vi "ConvertTextBasedCodeToLabVIEW_CreateClasses.vi"(0 "Classes":T11[](array[typedef])=[{"ClassName"="Program", "AccessScope"=enum."public", "Modifiers"=[], "ClassDocumentation"="", "Methods"=[{"ReturnType"={"Name"="", "DataType"=enum."void", "ArrayDim"=0, "CtrlPath"=path "", "DataTypeString"="void", "AccessScope"=enum."public", "InitialData"=variant(string "")}, "MethodName"="Main", "AccessScope"=enum."public", "Modifiers"=[enum."static"], "MethodDocumentation"="", "MethodContent"="public static void Main(string[] args)\n        {\n            // Create a subject and the observable, inject the subject into the observable\n            Subject subject = new Subject();\n            SubjectObservable observable = new SubjectObservable(subject);\n\n            //Create two observers\n            SubjectObserver zeus = new SubjectObserver(observable, \"Zeus\");\n            SubjectObserver ares = new SubjectObserver(observable, \"Ares\");\n            \n            // Run a loop and trigger the observer\n            for (int i = 0; i < 5; i++)\n            {\n                Console.WriteLine(\"Counter: \" + subject.Counter);\n                observable.inspectSubject();\n\n            }\n\n            Console.ReadLine();\n        }", "MethodArguments"=[{"Name"="args", "DataType"=enum."STRING", "ArrayDim"=1, "CtrlPath"=path "", "DataTypeString"="string[]", "AccessScope"=enum."public", "InitialData"=variant(string "")}], "GetProperty"={"Active"=FALSE, "AccessScope"=enum."public", "Code"=""}, "SetProperty"={"Active"=FALSE, "AccessScope"=enum."public", "Code"=""}}], "ParentClasses"=[], "ClassType"=enum."Class", "Owner"="Test", "OwnerType"=enum."Package/NameSpace", "Generics"=[], "Attributes"=[{"Name"="MyUINT8", "DataType"=enum."UINT8", "ArrayDim"=0, "CtrlPath"=path "", "DataTypeString"="", "AccessScope"=enum."public", "InitialData"=variant}], "Enums"=[{"Name"="MyEnum", "AccessScope"=enum."public", "Modifiers"=[], "Items"=["A1", "A2"], "Documentation"="My Enum Doc"}], "Structs"=[{"Name"="MyStruct", "AccessScope"=enum."public", "Modifiers"=[], "Items"=[{"Name"="MyObject", "DataType"=enum."LabVIEW Class", "ArrayDim"=1, "CtrlPath"=path "", "DataTypeString"="Program", "AccessScope"=enum."public", "InitialData"=variant}, {"Name"="Sträng", "DataType"=enum."STRING", "ArrayDim"=0, "CtrlPath"=path "", "DataTypeString"="", "AccessScope"=enum."public", "InitialData"=variant}], "Documentation"="Struct Doc"}]}, {"ClassName"="Subject", "AccessScope"=enum."public", "Modifiers"=[], "ClassDocumentation"="Class Subject - It has a counter object that increases everytime you inspect it", "Methods"=[{"ReturnType"={"Name"="", "DataType"=enum."INT32", "ArrayDim"=0, "CtrlPath"=path "", "DataTypeString"="int", "AccessScope"=enum."public", "InitialData"=variant(string "")}, "MethodName"="Counter", "AccessScope"=enum."public", "Modifiers"=[], "MethodDocumentation"="", "MethodContent"="public int Counter\n        {\n            get\n            {\n                return ++_counter;\n            }\n        }", "MethodArguments"=[], "GetProperty"={"Active"=TRUE, "AccessScope"=enum."public", "Code"="return ++_counter;"}, "SetProperty"={"Active"=FALSE, "AccessScope"=enum."public", "Code"=""}}], "ParentClasses"=[], "ClassType"=enum."Class", "Owner"="Test", "OwnerType"=enum."Package/NameSpace", "Generics"=[], "Attributes"=[{"Name"="_counter", "DataType"=enum."INT32", "ArrayDim"=0, "CtrlPath"=path "", "DataTypeString"="int", "AccessScope"=enum."private", "InitialData"=variant(string "")}], "Enums"=[], "Structs"=[]}, {"ClassName"="SubjectObservable", "AccessScope"=enum."public", "Modifiers"=[], "ClassDocumentation"="Class Subject Observable - The observable object that observes the subject and notifies the observers", "Methods"=[{"ReturnType"={"Name"="", "DataType"=enum."LabVIEW Object", "ArrayDim"=0, "CtrlPath"=path "", "DataTypeString"="SubjectObservable", "AccessScope"=enum."public", "InitialData"=variant(string "")}, "MethodName"="SubjectObservable", "AccessScope"=enum."public", "Modifiers"=[], "MethodDocumentation"="Accept a subject instance which we shall observe", "MethodContent"="public SubjectObservable(Subject subject)\n        {\n            _subjectObservers = new List<IObserver<Subject>>();\n            _subject = subject;\n\n        }", "MethodArguments"=[{"Name"="subject", "DataType"=enum."LabVIEW Object", "ArrayDim"=0, "CtrlPath"=path "", "DataTypeString"="Subject", "AccessScope"=enum."public", "InitialData"=variant(string "")}], "GetProperty"={"Active"=FALSE, "AccessScope"=enum."public", "Code"=""}, "SetProperty"={"Active"=FALSE, "AccessScope"=enum."public", "Code"=""}}, {"ReturnType"={"Name"="", "DataType"=enum."Other", "ArrayDim"=0, "CtrlPath"=path "", "DataTypeString"="IDisposable", "AccessScope"=enum."public", "InitialData"=variant(string "")}, "MethodName"="Subscribe", "AccessScope"=enum."public", "Modifiers"=[], "MethodDocumentation"="This method allows the observers to attach themselves. It returns a disposer object to the observer\nwhich the observer can utilize to unsubscribe", "MethodContent"="public IDisposable Subscribe(IObserver<Subject> observer)\n        {\n            if (!_subjectObservers.Contains(observer))\n            {\n                _subjectObservers.Add(observer);\n            }\n\n            return new Disposer(_subjectObservers, observer);\n        }", "MethodArguments"=[{"Name"="observer", "DataType"=enum."Other", "ArrayDim"=0, "CtrlPath"=path "", "DataTypeString"="IObserver<Subject>", "AccessScope"=enum."public", "InitialData"=variant(string "")}], "GetProperty"={"Active"=FALSE, "AccessScope"=enum."public", "Code"=""}, "SetProperty"={"Active"=FALSE, "AccessScope"=enum."public", "Code"=""}}, {"ReturnType"={"Name"="", "DataType"=enum."void", "ArrayDim"=0, "CtrlPath"=path "", "DataTypeString"="void", "AccessScope"=enum."public", "InitialData"=variant(string "")}, "MethodName"="inspectSubject", "AccessScope"=enum."public", "Modifiers"=[enum."event"], "MethodDocumentation"="This method is used to inspect the subject over time. Usually used with a timer or an event", "MethodContent"="event\n        public void inspectSubject()\n        {\n            foreach (IObserver<Subject> observer in _subjectObservers)\n            {\n                observer.OnNext(_subject);\n            }\n        }", "MethodArguments"=[], "GetProperty"={"Active"=FALSE, "AccessScope"=enum."public", "Code"=""}, "SetProperty"={"Active"=FALSE, "AccessScope"=enum."public", "Code"=""}}], "ParentClasses"=[{"ClassName"="IObservable", "ClassType"=enum."Undefined"}], "ClassType"=enum."Class", "Owner"="Test", "OwnerType"=enum."Package/NameSpace", "Generics"=["Subject"], "Attributes"=[{"Name"="_subjectObservers", "DataType"=enum."Other", "ArrayDim"=1, "CtrlPath"=path "", "DataTypeString"="IObserver<Subject>", "AccessScope"=enum."private", "InitialData"=variant(string "")}, {"Name"="_subject", "DataType"=enum."LabVIEW Object", "ArrayDim"=0, "CtrlPath"=path "", "DataTypeString"="Subject", "AccessScope"=enum."private", "InitialData"=variant(string "")}], "Enums"=[], "Structs"=[]}, {"ClassName"="SubjectObserver", "AccessScope"=enum."public", "Modifiers"=[], "ClassDocumentation"="Class Subject Observer - The object that attaches itself to a observable and recieves notifications", "Methods"=[{"ReturnType"={"Name"="", "DataType"=enum."LabVIEW Object", "ArrayDim"=0, "CtrlPath"=path "", "DataTypeString"="SubjectObserver", "AccessScope"=enum."public", "InitialData"=variant(string "")}, "MethodName"="SubjectObserver", "AccessScope"=enum."public", "Modifiers"=[], "MethodDocumentation"="", "MethodContent"="public SubjectObserver(IObservable<Subject> provider, string instanceName)\n        {\n            if (provider != null)\n            {\n                _disposer = provider.Subscribe(this);\n                _instaceName = instanceName;\n            }\n        }", "MethodArguments"=[{"Name"="provider", "DataType"=enum."Other", "ArrayDim"=0, "CtrlPath"=path "", "DataTypeString"="IObservable<Subject>", "AccessScope"=enum."public", "InitialData"=variant(string "")}, {"Name"="instanceName", "DataType"=enum."STRING", "ArrayDim"=0, "CtrlPath"=path "", "DataTypeString"="string", "AccessScope"=enum."public", "InitialData"=variant(string "")}], "GetProperty"={"Active"=FALSE, "AccessScope"=enum."public", "Code"=""}, "SetProperty"={"Active"=FALSE, "AccessScope"=enum."public", "Code"=""}}, {"ReturnType"={"Name"="", "DataType"=enum."void", "ArrayDim"=0, "CtrlPath"=path "", "DataTypeString"="void", "AccessScope"=enum."public", "InitialData"=variant(string "")}, "MethodName"="OnNext", "AccessScope"=enum."public", "Modifiers"=[], "MethodDocumentation"="The observable invokes this method to pass the Subject object to the observer", "MethodContent"="public void OnNext(Subject value)\n        {\n            Console.WriteLine(\"[\" + _instaceName + \"] \" + value.Counter);\n        }", "MethodArguments"=[{"Name"="value", "DataType"=enum."LabVIEW Object", "ArrayDim"=0, "CtrlPath"=path "", "DataTypeString"="Subject", "AccessScope"=enum."public", "InitialData"=variant(string "")}], "GetProperty"={"Active"=FALSE, "AccessScope"=enum."public", "Code"=""}, "SetProperty"={"Active"=FALSE, "AccessScope"=enum."public", "Code"=""}}, {"ReturnType"={"Name"="", "DataType"=enum."void", "ArrayDim"=0, "CtrlPath"=path "", "DataTypeString"="void", "AccessScope"=enum."public", "InitialData"=variant(string "")}, "MethodName"="OnCompleted", "AccessScope"=enum."public", "Modifiers"=[], "MethodDocumentation"="Usually called when a transmission is complete. Not implemented.", "MethodContent"="public void OnCompleted()\n        {\n            throw new NotImplementedException();\n        }", "MethodArguments"=[], "GetProperty"={"Active"=FALSE, "AccessScope"=enum."public", "Code"=""}, "SetProperty"={"Active"=FALSE, "AccessScope"=enum."public", "Code"=""}}, {"ReturnType"={"Name"="", "DataType"=enum."void", "ArrayDim"=0, "CtrlPath"=path "", "DataTypeString"="void", "AccessScope"=enum."public", "InitialData"=variant(string "")}, "MethodName"="OnError", "AccessScope"=enum."public", "Modifiers"=[], "MethodDocumentation"="Usually called when there was an error. Didn't implement.", "MethodContent"="public void OnError(Exception error)\n        {\n            throw new NotImplementedException();\n        }", "MethodArguments"=[{"Name"="error", "DataType"=enum."Other", "ArrayDim"=0, "CtrlPath"=path "", "DataTypeString"="Exception", "AccessScope"=enum."public", "InitialData"=variant(string "")}], "GetProperty"={"Active"=FALSE, "AccessScope"=enum."public", "Code"=""}, "SetProperty"={"Active"=FALSE, "AccessScope"=enum."public", "Code"=""}}, {"ReturnType"={"Name"="", "DataType"=enum."void", "ArrayDim"=0, "CtrlPath"=path "", "DataTypeString"="void", "AccessScope"=enum."public", "InitialData"=variant(string "")}, "MethodName"="Dispose", "AccessScope"=enum."public", "Modifiers"=[], "MethodDocumentation"="Invoke the disposer recieved from the observable. This will unsubscribe", "MethodContent"="public void Dispose()\n        {\n            _disposer.Dispose();\n        }", "MethodArguments"=[], "GetProperty"={"Active"=FALSE, "AccessScope"=enum."public", "Code"=""}, "SetProperty"={"Active"=FALSE, "AccessScope"=enum."public", "Code"=""}}], "ParentClasses"=[{"ClassName"="IObserver", "ClassType"=enum."Undefined"}], "ClassType"=enum."Class", "Owner"="Test", "OwnerType"=enum."Package/NameSpace", "Generics"=["Subject"], "Attributes"=[{"Name"="_disposer", "DataType"=enum."Other", "ArrayDim"=0, "CtrlPath"=path "", "DataTypeString"="IDisposable", "AccessScope"=enum."private", "InitialData"=variant(string "")}, {"Name"="_instaceName", "DataType"=enum."STRING", "ArrayDim"=0, "CtrlPath"=path "", "DataTypeString"="string", "AccessScope"=enum."private", "InitialData"=variant(string "")}], "Enums"=[], "Structs"=[]}, {"ClassName"="Disposer", "AccessScope"=enum."private", "Modifiers"=[], "ClassDocumentation"="Private class Disposer: Implements the IDisposable. Observable returns an instance to the observer for easy unsubscription\nprivate", "Methods"=[{"ReturnType"={"Name"="", "DataType"=enum."LabVIEW Object", "ArrayDim"=0, "CtrlPath"=path "", "DataTypeString"="Disposer", "AccessScope"=enum."public", "InitialData"=variant(string "")}, "MethodName"="Disposer", "AccessScope"=enum."public", "Modifiers"=[], "MethodDocumentation"="", "MethodContent"="public Disposer(List<IObserver<Subject>> _subObservers, IObserver<Subject> observer)\n            {\n                _subjectObservers = _subObservers;\n                _observer = observer;\n            }", "MethodArguments"=[{"Name"="_subObservers", "DataType"=enum."Other", "ArrayDim"=1, "CtrlPath"=path "", "DataTypeString"="IObserver<Subject>", "AccessScope"=enum."public", "InitialData"=variant(string "")}, {"Name"="observer", "DataType"=enum."Other", "ArrayDim"=0, "CtrlPath"=path "", "DataTypeString"="IObserver<Subject>", "AccessScope"=enum."public", "InitialData"=variant(string "")}], "GetProperty"={"Active"=FALSE, "AccessScope"=enum."public", "Code"=""}, "SetProperty"={"Active"=FALSE, "AccessScope"=enum."public", "Code"=""}}, {"ReturnType"={"Name"="", "DataType"=enum."void", "ArrayDim"=0, "CtrlPath"=path "", "DataTypeString"="void", "AccessScope"=enum."public", "InitialData"=variant(string "")}, "MethodName"="Dispose", "AccessScope"=enum."public", "Modifiers"=[], "MethodDocumentation"="", "MethodContent"="public void Dispose()\n            {\n                if (_subjectObservers.Contains(_observer))\n                {\n                    _subjectObservers.Remove(_observer);\n                }\n            }", "MethodArguments"=[], "GetProperty"={"Active"=FALSE, "AccessScope"=enum."public", "Code"=""}, "SetProperty"={"Active"=FALSE, "AccessScope"=enum."public", "Code"=""}}], "ParentClasses"=[{"ClassName"="IDisposable", "ClassType"=enum."Undefined"}], "ClassType"=enum."Class", "Owner"="SubjectObservable", "OwnerType"=enum."Class", "Generics"=[], "Attributes"=[{"Name"="_subjectObservers", "DataType"=enum."Other", "ArrayDim"=1, "CtrlPath"=path "", "DataTypeString"="IObserver<Subject>", "AccessScope"=enum."private", "InitialData"=variant(string "")}, {"Name"="_observer", "DataType"=enum."Other", "ArrayDim"=0, "CtrlPath"=path "", "DataTypeString"="IObserver<Subject>", "AccessScope"=enum."private", "InitialData"=variant(string "")}], "Enums"=[], "Structs"=[]}], 1 "TopFolder":path=path "D:/Temp", 2 "InterfacesThatShouldBeConvertedToClasses":string[](array[string]), 3 "Options":T7={"ClassProvider"=enum."LabVIEW Native(By value)", "PropertyMethodType"=enum."PropertyMethod", "Pattern type"=2} {"Pattern type" items=["4x4x4", "5x6x5", "6x8x6"]}, 5 "MissingItems":T17[](array[typedef])=[{"Item"="IObservable", "Options"=["Select action to handle missing type", "Create stub code as class", "Create stub code as interface by VI Server", "Remove dependency to this type"], "Icons"=[enum."?", enum."Add", enum."Add", enum."Delete"], "Index"=2}, {"Item"="IDisposable", "Options"=["Select action to handle missing type", "Create stub code as class", "Create stub code as interface by VI Server", "Remove dependency to this type"], "Icons"=[enum."?", enum."Add", enum."Add", enum."Delete"], "Index"=1}, {"Item"="IObserver", "Options"=["Select action to handle missing type", "Create stub code as class", "Create stub code as interface by VI Server", "Remove dependency to this type"], "Icons"=[enum."?", enum."Add", enum."Add", enum."Delete"], "Index"=2}, {"Item"="Exception", "Options"=["Select action to handle missing type", "Create stub code as class", "Remove dependency to this type"], "Icons"=[enum."?", enum."Add", enum."Delete"], "Index"=2}], 7 "BetterNames":bool, 9 "ExistingClassFolders":path[](array[path]), 11 "error in (no error)":errorcluster, 12 "ProgressTextRef":refnum<vi>, 13 "StructsOusideClass":T1[](array[typedef]), 14 "EnumsOusideClass":T6[](array[typedef])) -> (15 "error out":errorcluster)   [LabVIEW 2016]
uses:
  <resource>/Framework/Providers/Open_GDS/ClassProviders/Common/ConvertTextToLv_SubVIs/ConvertTextBasedCodeToLabVIEW_MissingType.ctl
  <resource>/Framework/Providers/Open_GDS/ClassProviders/Common/ConvertTextToLv_SubVIs/ConvertTextBasedCodeToLabVIEW_MissingTypeIconType.ctl
  <resource>/Framework/Providers/Open_GDS/ClassProviders/Common/String/GDSString_ClassDescriptionType.ctl
  <resource>/Framework/Providers/Open_GDS/ClassProviders/Common/String/GDSString_AccessScopeModifierType.ctl
  <resource>/Framework/Providers/Open_GDS/ClassProviders/Common/String/GDSString_ModifierType.ctl
  <resource>/Framework/Providers/Open_GDS/ClassProviders/Common/String/GDSString_MethodDescriptionType.ctl
  <resource>/Framework/Providers/Open_GDS/ClassProviders/Common/CommonVIs/CommonVIs_AttributeType.ctl
  <resource>/Framework/Providers/Open_GDS/ClassProviders/Common/CommonVIs/CommonVIs_AttributeDataType.ctl
  <resource>/Framework/Providers/Open_GDS/ClassProviders/Common/CommonVIs/CommonVIs_PropertyType.ctl
  <resource>/Framework/Providers/Open_GDS/ClassProviders/Common/String/GDSString_ClassParentType.ctl
  <resource>/Framework/Providers/Open_GDS/ClassProviders/Common/String/GDSString_ClassType.ctl
  <resource>/Framework/Providers/Open_GDS/ClassProviders/Common/String/GDSString_ClassOwnerType.ctl
  <resource>/Framework/Providers/Open_GDS/ClassProviders/Common/CommonVIs/CommonVIs_EnumType.ctl
  <resource>/Framework/Providers/Open_GDS/ClassProviders/Common/CommonVIs/CommonVIs_StructType.ctl
  <resource>/Framework/Providers/Open_GDS/ClassProviders/Common/ConvertTextToLv_SubVIs/ConvertTextBasedCodeToLabVIEW_CreateClassesOption.ctl
  <resource>/Framework/Providers/Open_GDS/API/GDSAPI_SubVIs/GDSAPI_ClassProviderType.ctl
  <resource>/Framework/Providers/Open_GDS/API/GDSAPI_SubVIs/GDSAPI_PropertyMethodType.ctl
  <resource>/Framework/Providers/Open_GDS/ClassProviders/Common/ScriptingFunctions/Scripting_ConnectorPanePatternType.ctl
  <resource>/Framework/Providers/Open_GDS/ClassProviders/Common/CommonVIs/CommonVIs_ClassNamePathType.ctl
  <resource>/Framework/Providers/Open_GDS/API/GDSAPI_SubVIs/GDSAPI_SetClassOptionsAction.ctl
  <resource>/Framework/Providers/Open_GDS/ClassProviders/Common/ConvertTextToLv_SubVIs/ConvertTextBasedCodeToLabVIEW_MissingTypeOptions.ctl
  <resource>/Framework/Providers/Open_GDS/API/GDSAPI_CreateClassType.ctl
  <resource>/Framework/Providers/Open_GDS/API/GDSAPI_SubVIs/GDSAPI_ClassTemplateType.ctl
  <resource>/Framework/Providers/Open_GDS/API/GDSAPI_SubVIs/GDSAPI_ProjectIconType.ctl
panel:
  out "ClassesOut":T11[](array[typedef])=[{"ClassName"="Program", "AccessScope"=enum."public", "Modifiers"=[], "ClassDocumentation"="", "Methods"=[{"ReturnType"={"Name"="", "DataType"=enum."void", "ArrayDim"=0, "CtrlPath"=path "", "DataTypeString"="void", "AccessScope"=enum."public", "InitialData"=variant(string "")}, "MethodName"="Main", "AccessScope"=enum."public", "Modifiers"=[enum."static"], "MethodDocumentation"="", "MethodContent"="public static void Main(string[] args)\n        {\n            // Create a subject and the observable, inject the subject into the observable\n            Subject subject = new Subject();\n            SubjectObservable observable = new SubjectObservable(subject);\n\n            //Create two observers\n            SubjectObserver zeus = new SubjectObserver(observable, \"Zeus\");\n            SubjectObserver ares = new SubjectObserver(observable, \"Ares\");\n            \n            // Run a loop and trigger the observer\n            for (int i = 0; i < 5; i++)\n            {\n                Console.WriteLine(\"Counter: \" + subject.Counter);\n                observable.inspectSubject();\n\n            }\n\n            Console.ReadLine();\n        }", "MethodArguments"=[{"Name"="args", "DataType"=enum."STRING", "ArrayDim"=1, "CtrlPath"=path "", "DataTypeString"="string[]", "AccessScope"=enum."public", "InitialData"=variant(string "")}], "GetProperty"={"Active"=FALSE, "AccessScope"=enum."public", "Code"=""}, "SetProperty"={"Active"=FALSE, "AccessScope"=enum."public", "Code"=""}}], "ParentClasses"=[], "ClassType"=enum."Class", "Owner"="Test", "OwnerType"=enum."Package/NameSpace", "Generics"=[], "Attributes"=[{"Name"="MyUINT8", "DataType"=enum."UINT8", "ArrayDim"=0, "CtrlPath"=path "", "DataTypeString"="", "AccessScope"=enum."public", "InitialData"=variant}], "Enums"=[{"Name"="MyEnum", "AccessScope"=enum."public", "Modifiers"=[], "Items"=["A1", "A2"], "Documentation"="My Enum Doc"}], "Structs"=[{"Name"="MyStruct", "AccessScope"=enum."public", "Modifiers"=[], "Items"=[{"Name"="MyObject", "DataType"=enum."LabVIEW Class", "ArrayDim"=1, "CtrlPath"=path "", "DataTypeString"="Program", "AccessScope"=enum."public", "InitialData"=variant}, {"Name"="Sträng", "DataType"=enum."STRING", "ArrayDim"=0, "CtrlPath"=path "", "DataTypeString"="", "AccessScope"=enum."public", "InitialData"=variant}], "Documentation"="Struct Doc"}]}, {"ClassName"="Subject", "AccessScope"=enum."public", "Modifiers"=[], "ClassDocumentation"="Class Subject - It has a counter object that increases everytime you inspect it", "Methods"=[{"ReturnType"={"Name"="", "DataType"=enum."INT32", "ArrayDim"=0, "CtrlPath"=path "", "DataTypeString"="int", "AccessScope"=enum."public", "InitialData"=variant(string "")}, "MethodName"="Counter", "AccessScope"=enum."public", "Modifiers"=[], "MethodDocumentation"="", "MethodContent"="public int Counter\n        {\n            get\n            {\n                return ++_counter;\n            }\n        }", "MethodArguments"=[], "GetProperty"={"Active"=TRUE, "AccessScope"=enum."public", "Code"="return ++_counter;"}, "SetProperty"={"Active"=FALSE, "AccessScope"=enum."public", "Code"=""}}], "ParentClasses"=[], "ClassType"=enum."Class", "Owner"="Test", "OwnerType"=enum."Package/NameSpace", "Generics"=[], "Attributes"=[{"Name"="_counter", "DataType"=enum."INT32", "ArrayDim"=0, "CtrlPath"=path "", "DataTypeString"="int", "AccessScope"=enum."private", "InitialData"=variant(string "")}], "Enums"=[], "Structs"=[]}, {"ClassName"="SubjectObservable", "AccessScope"=enum."public", "Modifiers"=[], "ClassDocumentation"="Class Subject Observable - The observable object that observes the subject and notifies the observers", "Methods"=[{"ReturnType"={"Name"="", "DataType"=enum."LabVIEW Object", "ArrayDim"=0, "CtrlPath"=path "", "DataTypeString"="SubjectObservable", "AccessScope"=enum."public", "InitialData"=variant(string "")}, "MethodName"="SubjectObservable", "AccessScope"=enum."public", "Modifiers"=[], "MethodDocumentation"="Accept a subject instance which we shall observe", "MethodContent"="public SubjectObservable(Subject subject)\n        {\n            _subjectObservers = new List<IObserver<Subject>>();\n            _subject = subject;\n\n        }", "MethodArguments"=[{"Name"="subject", "DataType"=enum."LabVIEW Object", "ArrayDim"=0, "CtrlPath"=path "", "DataTypeString"="Subject", "AccessScope"=enum."public", "InitialData"=variant(string "")}], "GetProperty"={"Active"=FALSE, "AccessScope"=enum."public", "Code"=""}, "SetProperty"={"Active"=FALSE, "AccessScope"=enum."public", "Code"=""}}, {"ReturnType"={"Name"="", "DataType"=enum."Other", "ArrayDim"=0, "CtrlPath"=path "", "DataTypeString"="IDisposable", "AccessScope"=enum."public", "InitialData"=variant(string "")}, "MethodName"="Subscribe", "AccessScope"=enum."public", "Modifiers"=[], "MethodDocumentation"="This method allows the observers to attach themselves. It returns a disposer object to the observer\nwhich the observer can utilize to unsubscribe", "MethodContent"="public IDisposable Subscribe(IObserver<Subject> observer)\n        {\n            if (!_subjectObservers.Contains(observer))\n            {\n                _subjectObservers.Add(observer);\n            }\n\n            return new Disposer(_subjectObservers, observer);\n        }", "MethodArguments"=[{"Name"="observer", "DataType"=enum."Other", "ArrayDim"=0, "CtrlPath"=path "", "DataTypeString"="IObserver<Subject>", "AccessScope"=enum."public", "InitialData"=variant(string "")}], "GetProperty"={"Active"=FALSE, "AccessScope"=enum."public", "Code"=""}, "SetProperty"={"Active"=FALSE, "AccessScope"=enum."public", "Code"=""}}, {"ReturnType"={"Name"="", "DataType"=enum."void", "ArrayDim"=0, "CtrlPath"=path "", "DataTypeString"="void", "AccessScope"=enum."public", "InitialData"=variant(string "")}, "MethodName"="inspectSubject", "AccessScope"=enum."public", "Modifiers"=[enum."event"], "MethodDocumentation"="This method is used to inspect the subject over time. Usually used with a timer or an event", "MethodContent"="event\n        public void inspectSubject()\n        {\n            foreach (IObserver<Subject> observer in _subjectObservers)\n            {\n                observer.OnNext(_subject);\n            }\n        }", "MethodArguments"=[], "GetProperty"={"Active"=FALSE, "AccessScope"=enum."public", "Code"=""}, "SetProperty"={"Active"=FALSE, "AccessScope"=enum."public", "Code"=""}}], "ParentClasses"=[{"ClassName"="IObservable", "ClassType"=enum."Undefined"}], "ClassType"=enum."Class", "Owner"="Test", "OwnerType"=enum."Package/NameSpace", "Generics"=["Subject"], "Attributes"=[{"Name"="_subjectObservers", "DataType"=enum."Other", "ArrayDim"=1, "CtrlPath"=path "", "DataTypeString"="IObserver<Subject>", "AccessScope"=enum."private", "InitialData"=variant(string "")}, {"Name"="_subject", "DataType"=enum."LabVIEW Object", "ArrayDim"=0, "CtrlPath"=path "", "DataTypeString"="Subject", "AccessScope"=enum."private", "InitialData"=variant(string "")}], "Enums"=[], "Structs"=[]}, {"ClassName"="SubjectObserver", "AccessScope"=enum."public", "Modifiers"=[], "ClassDocumentation"="Class Subject Observer - The object that attaches itself to a observable and recieves notifications", "Methods"=[{"ReturnType"={"Name"="", "DataType"=enum."LabVIEW Object", "ArrayDim"=0, "CtrlPath"=path "", "DataTypeString"="SubjectObserver", "AccessScope"=enum."public", "InitialData"=variant(string "")}, "MethodName"="SubjectObserver", "AccessScope"=enum."public", "Modifiers"=[], "MethodDocumentation"="", "MethodContent"="public SubjectObserver(IObservable<Subject> provider, string instanceName)\n        {\n            if (provider != null)\n            {\n                _disposer = provider.Subscribe(this);\n                _instaceName = instanceName;\n            }\n        }", "MethodArguments"=[{"Name"="provider", "DataType"=enum."Other", "ArrayDim"=0, "CtrlPath"=path "", "DataTypeString"="IObservable<Subject>", "AccessScope"=enum."public", "InitialData"=variant(string "")}, {"Name"="instanceName", "DataType"=enum."STRING", "ArrayDim"=0, "CtrlPath"=path "", "DataTypeString"="string", "AccessScope"=enum."public", "InitialData"=variant(string "")}], "GetProperty"={"Active"=FALSE, "AccessScope"=enum."public", "Code"=""}, "SetProperty"={"Active"=FALSE, "AccessScope"=enum."public", "Code"=""}}, {"ReturnType"={"Name"="", "DataType"=enum."void", "ArrayDim"=0, "CtrlPath"=path "", "DataTypeString"="void", "AccessScope"=enum."public", "InitialData"=variant(string "")}, "MethodName"="OnNext", "AccessScope"=enum."public", "Modifiers"=[], "MethodDocumentation"="The observable invokes this method to pass the Subject object to the observer", "MethodContent"="public void OnNext(Subject value)\n        {\n            Console.WriteLine(\"[\" + _instaceName + \"] \" + value.Counter);\n        }", "MethodArguments"=[{"Name"="value", "DataType"=enum."LabVIEW Object", "ArrayDim"=0, "CtrlPath"=path "", "DataTypeString"="Subject", "AccessScope"=enum."public", "InitialData"=variant(string "")}], "GetProperty"={"Active"=FALSE, "AccessScope"=enum."public", "Code"=""}, "SetProperty"={"Active"=FALSE, "AccessScope"=enum."public", "Code"=""}}, {"ReturnType"={"Name"="", "DataType"=enum."void", "ArrayDim"=0, "CtrlPath"=path "", "DataTypeString"="void", "AccessScope"=enum."public", "InitialData"=variant(string "")}, "MethodName"="OnCompleted", "AccessScope"=enum."public", "Modifiers"=[], "MethodDocumentation"="Usually called when a transmission is complete. Not implemented.", "MethodContent"="public void OnCompleted()\n        {\n            throw new NotImplementedException();\n        }", "MethodArguments"=[], "GetProperty"={"Active"=FALSE, "AccessScope"=enum."public", "Code"=""}, "SetProperty"={"Active"=FALSE, "AccessScope"=enum."public", "Code"=""}}, {"ReturnType"={"Name"="", "DataType"=enum."void", "ArrayDim"=0, "CtrlPath"=path "", "DataTypeString"="void", "AccessScope"=enum."public", "InitialData"=variant(string "")}, "MethodName"="OnError", "AccessScope"=enum."public", "Modifiers"=[], "MethodDocumentation"="Usually called when there was an error. Didn't implement.", "MethodContent"="public void OnError(Exception error)\n        {\n            throw new NotImplementedException();\n        }", "MethodArguments"=[{"Name"="error", "DataType"=enum."Other", "ArrayDim"=0, "CtrlPath"=path "", "DataTypeString"="Exception", "AccessScope"=enum."public", "InitialData"=variant(string "")}], "GetProperty"={"Active"=FALSE, "AccessScope"=enum."public", "Code"=""}, "SetProperty"={"Active"=FALSE, "AccessScope"=enum."public", "Code"=""}}, {"ReturnType"={"Name"="", "DataType"=enum."void", "ArrayDim"=0, "CtrlPath"=path "", "DataTypeString"="void", "AccessScope"=enum."public", "InitialData"=variant(string "")}, "MethodName"="Dispose", "AccessScope"=enum."public", "Modifiers"=[], "MethodDocumentation"="Invoke the disposer recieved from the observable. This will unsubscribe", "MethodContent"="public void Dispose()\n        {\n            _disposer.Dispose();\n        }", "MethodArguments"=[], "GetProperty"={"Active"=FALSE, "AccessScope"=enum."public", "Code"=""}, "SetProperty"={"Active"=FALSE, "AccessScope"=enum."public", "Code"=""}}], "ParentClasses"=[{"ClassName"="IObserver", "ClassType"=enum."Undefined"}], "ClassType"=enum."Class", "Owner"="Test", "OwnerType"=enum."Package/NameSpace", "Generics"=["Subject"], "Attributes"=[{"Name"="_disposer", "DataType"=enum."Other", "ArrayDim"=0, "CtrlPath"=path "", "DataTypeString"="IDisposable", "AccessScope"=enum."private", "InitialData"=variant(string "")}, {"Name"="_instaceName", "DataType"=enum."STRING", "ArrayDim"=0, "CtrlPath"=path "", "DataTypeString"="string", "AccessScope"=enum."private", "InitialData"=variant(string "")}], "Enums"=[], "Structs"=[]}, {"ClassName"="Disposer", "AccessScope"=enum."private", "Modifiers"=[], "ClassDocumentation"="Private class Disposer: Implements the IDisposable. Observable returns an instance to the observer for easy unsubscription\nprivate", "Methods"=[{"ReturnType"={"Name"="", "DataType"=enum."LabVIEW Object", "ArrayDim"=0, "CtrlPath"=path "", "DataTypeString"="Disposer", "AccessScope"=enum."public", "InitialData"=variant(string "")}, "MethodName"="Disposer", "AccessScope"=enum."public", "Modifiers"=[], "MethodDocumentation"="", "MethodContent"="public Disposer(List<IObserver<Subject>> _subObservers, IObserver<Subject> observer)\n            {\n                _subjectObservers = _subObservers;\n                _observer = observer;\n            }", "MethodArguments"=[{"Name"="_subObservers", "DataType"=enum."Other", "ArrayDim"=1, "CtrlPath"=path "", "DataTypeString"="IObserver<Subject>", "AccessScope"=enum."public", "InitialData"=variant(string "")}, {"Name"="observer", "DataType"=enum."Other", "ArrayDim"=0, "CtrlPath"=path "", "DataTypeString"="IObserver<Subject>", "AccessScope"=enum."public", "InitialData"=variant(string "")}], "GetProperty"={"Active"=FALSE, "AccessScope"=enum."public", "Code"=""}, "SetProperty"={"Active"=FALSE, "AccessScope"=enum."public", "Code"=""}}, {"ReturnType"={"Name"="", "DataType"=enum."void", "ArrayDim"=0, "CtrlPath"=path "", "DataTypeString"="void", "AccessScope"=enum."public", "InitialData"=variant(string "")}, "MethodName"="Dispose", "AccessScope"=enum."public", "Modifiers"=[], "MethodDocumentation"="", "MethodContent"="public void Dispose()\n            {\n                if (_subjectObservers.Contains(_observer))\n                {\n                    _subjectObservers.Remove(_observer);\n                }\n            }", "MethodArguments"=[], "GetProperty"={"Active"=FALSE, "AccessScope"=enum."public", "Code"=""}, "SetProperty"={"Active"=FALSE, "AccessScope"=enum."public", "Code"=""}}], "ParentClasses"=[{"ClassName"="IDisposable", "ClassType"=enum."Undefined"}], "ClassType"=enum."Class", "Owner"="SubjectObservable", "OwnerType"=enum."Class", "Generics"=[], "Attributes"=[{"Name"="_subjectObservers", "DataType"=enum."Other", "ArrayDim"=1, "CtrlPath"=path "", "DataTypeString"="IObserver<Subject>", "AccessScope"=enum."private", "InitialData"=variant(string "")}, {"Name"="_observer", "DataType"=enum."Other", "ArrayDim"=0, "CtrlPath"=path "", "DataTypeString"="IObserver<Subject>", "AccessScope"=enum."private", "InitialData"=variant(string "")}], "Enums"=[], "Structs"=[]}]
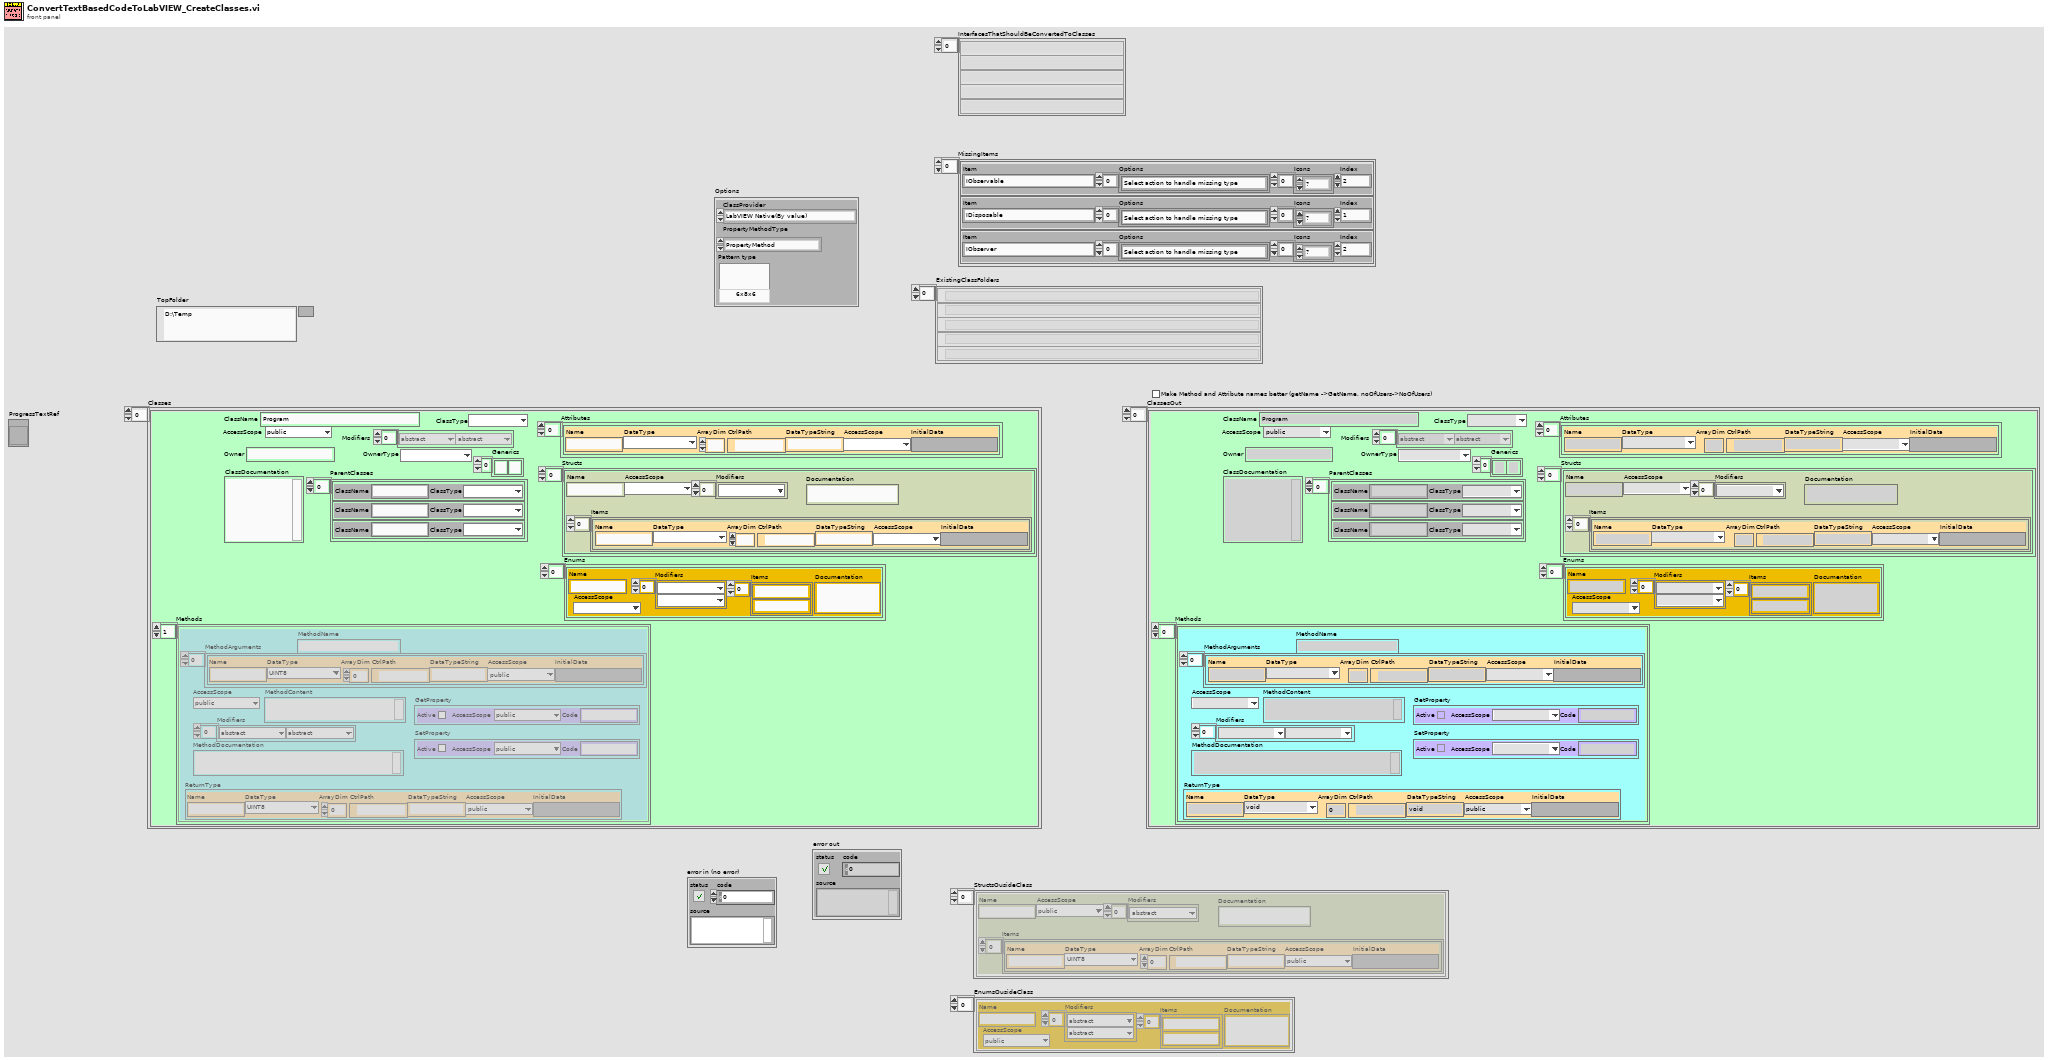
[diagram p1: front panel]
types:
  T1 = typedef "CommonVIs_StructType.ctl" = cluster{"Name":string, "AccessScope":T2, "Modifiers":T3[], "Items":T4[], "Documentation":string}
  T2 = typedef "GDSString_AccessScopeModifierType.ctl" = enum16{"public", "private", "protected", "internal"}
  T3 = typedef "GDSString_ModifierType.ctl" = enum16{"abstract", "static", "final", "synchronized", "strictfp", "async", "const", "event", "extern", "new", "native ", "override", "partial", "readonly", "sealed", "unsafe", "virtual", "volatile"}
  T4 = typedef "CommonVIs_AttributeType.ctl" = cluster{"Name":string, "DataType":T5, "ArrayDim":i32, "CtrlPath":path, "DataTypeString":string, "AccessScope":T2, "InitialData":variant}
  T5 = typedef "CommonVIs_AttributeDataType.ctl" = enum16{"UINT8", "INT8", "UINT16", "INT16", "UINT32", "INT32", "UINT64", "INT64", "SGL", "DBL", "EXT", "CSG", "CDB", "CXT", "TimeStamp", "STRING", "PATH", "BOOL", "ENUM", "RefNum", "VIRefNum", "LabVIEW Class", "Cluster", "Variant", "TypeDef", "Waveform", "LabVIEW Object", "Other", "void"}
  T6 = typedef "CommonVIs_EnumType.ctl" = cluster{"Name":string, "AccessScope":T2, "Modifiers":T3[], "Items":string[], "Documentation":string}
  T7 = typedef "ConvertTextBasedCodeToLabVIEW_CreateClassesOption.ctl" = cluster{"ClassProvider":T8, "PropertyMethodType":T9, "Pattern type":T10}
  T8 = typedef "GDSAPI_ClassProviderType.ctl" = enum16{"LabVIEW Native(By value)", "GOOP-3(By reference)", "GOOP-4(By reference)"}
  T9 = typedef "GDSAPI_PropertyMethodType.ctl" = enum16{"PropertyMethod", "PropertyNode"}
  T10 = typedef "Scripting_ConnectorPanePatternType.ctl" = u16
  T11 = typedef "GDSString_ClassDescriptionType.ctl" = cluster{"ClassName":string, "AccessScope":T2, "Modifiers":T3[], "ClassDocumentation":string, "Methods":T12[], "ParentClasses":T14[], "ClassType":T15, "Owner":string, "OwnerType":T16, "Generics":string[], "Attributes":T4[], "Enums":T6[], "Structs":T1[]}
  T12 = typedef "GDSString_MethodDescriptionType.ctl" = cluster{"ReturnType":T4, "MethodName":string, "AccessScope":T2, "Modifiers":T3[], "MethodDocumentation":string, "MethodContent":string, "MethodArguments":T4[], "GetProperty":T13, "SetProperty":T13}
  T13 = typedef "CommonVIs_PropertyType.ctl" = cluster{"Active":bool, "AccessScope":T2, "Code":string}
  T14 = typedef "GDSString_ClassParentType.ctl" = cluster{"ClassName":string, "ClassType":T15}
  T15 = typedef "GDSString_ClassType.ctl" = enum16{"Undefined", "Class", "Interface"}
  T16 = typedef "GDSString_ClassOwnerType.ctl" = enum16{"NoOwner", "Class", "Package/NameSpace"}
  T17 = typedef "ConvertTextBasedCodeToLabVIEW_MissingType.ctl" = cluster{"Item":string, "Options":string[], "Icons":T18[], "Index":i32}
  T18 = typedef "ConvertTextBasedCodeToLabVIEW_MissingTypeIconType.ctl" = enum16{"?", "Add", "Delete", "Implement", "Inherit"}
  T19 = typedef "GDSAPI_SetClassOptionsAction.ctl" = enum16{"Set All", "Set Project Icon Type", "Set Pattern Type", "Set Wire Configuration"}
  T20 = typedef "CommonVIs_ClassNamePathType.ctl" = cluster{"ClassNamn":string, "ClassPath":path, "InterfaceClass":bool}
  T21 = cluster{"App":refnum<vi>, "Proj":refnum<vi>, "ClassesToCreate":string[], "StructsToCreate":string[], "EnumsToCreate":string[], "Classes":T11[], "ProjItem":refnum<vi>, "ClassPath":path[], "ExistingClasses/Types":string[], "ClassRefs":refnum<vi>[], "ClassInfo":T20[], "StartTime":timestamp, "MissingTypes":string[], "Pattern-Before":T10, "ClassesStart":T11[]}
  T22 = typedef "ConvertTextBasedCodeToLabVIEW_MissingTypeOptions.ctl" = enum16{"Select action to handle missing type", "Create stub code as class", "Create stub code as interface by VI Server", "Remove dependency to this type"}
  T23 = typedef "GDSAPI_CreateClassType.ctl" = cluster{"ClassProvider":T8, "NewClassFolder":path, "ParentLvClassFilePath":path, "ClassName":string, "ClassDescription":string, "ClassTemplate":T24}
  T24 = typedef "GDSAPI_ClassTemplateType.ctl" = enum16{"Standard", "Singleton", "Interface(By Aggregation)", "Interface(By VI Server)"}
  T25 = typedef "GDSAPI_ProjectIconType.ctl" = enum16{"BlueCircle", "BlueFrame", "BlueFull", "BlueMessage", "BrownCircle", "BrownFrame", "BrownFull", "BurgundyCircle", "BurgundyFrame", "BurgundyFull", "CyanCircle", "CyanFrame", "CyanFull", "DarkBlueCircle", "DarkBlueFrame", "DarkBlueFull", "ForestGreenCircle", "ForestGreenFrame", "ForestGreenFull", "GrayCircle", "GrayFrame", "GrayFull", "GreenCircle", "GreenFrame", "GreenFull", "LightGreenCircle", "LightGreenFrame", "LightGreenFull", "LightRedCircle", "LightRedFrame", "LightRedFull", "PinkCircle", "PinkFrame", "PinkFull", "PurpleCircle", "PurpleFrame", "PurpleFull", "RedCircle", "RedFrame", "RedFull", "YellowCircle", "YellowFrame", "YellowFull", "Interface"}
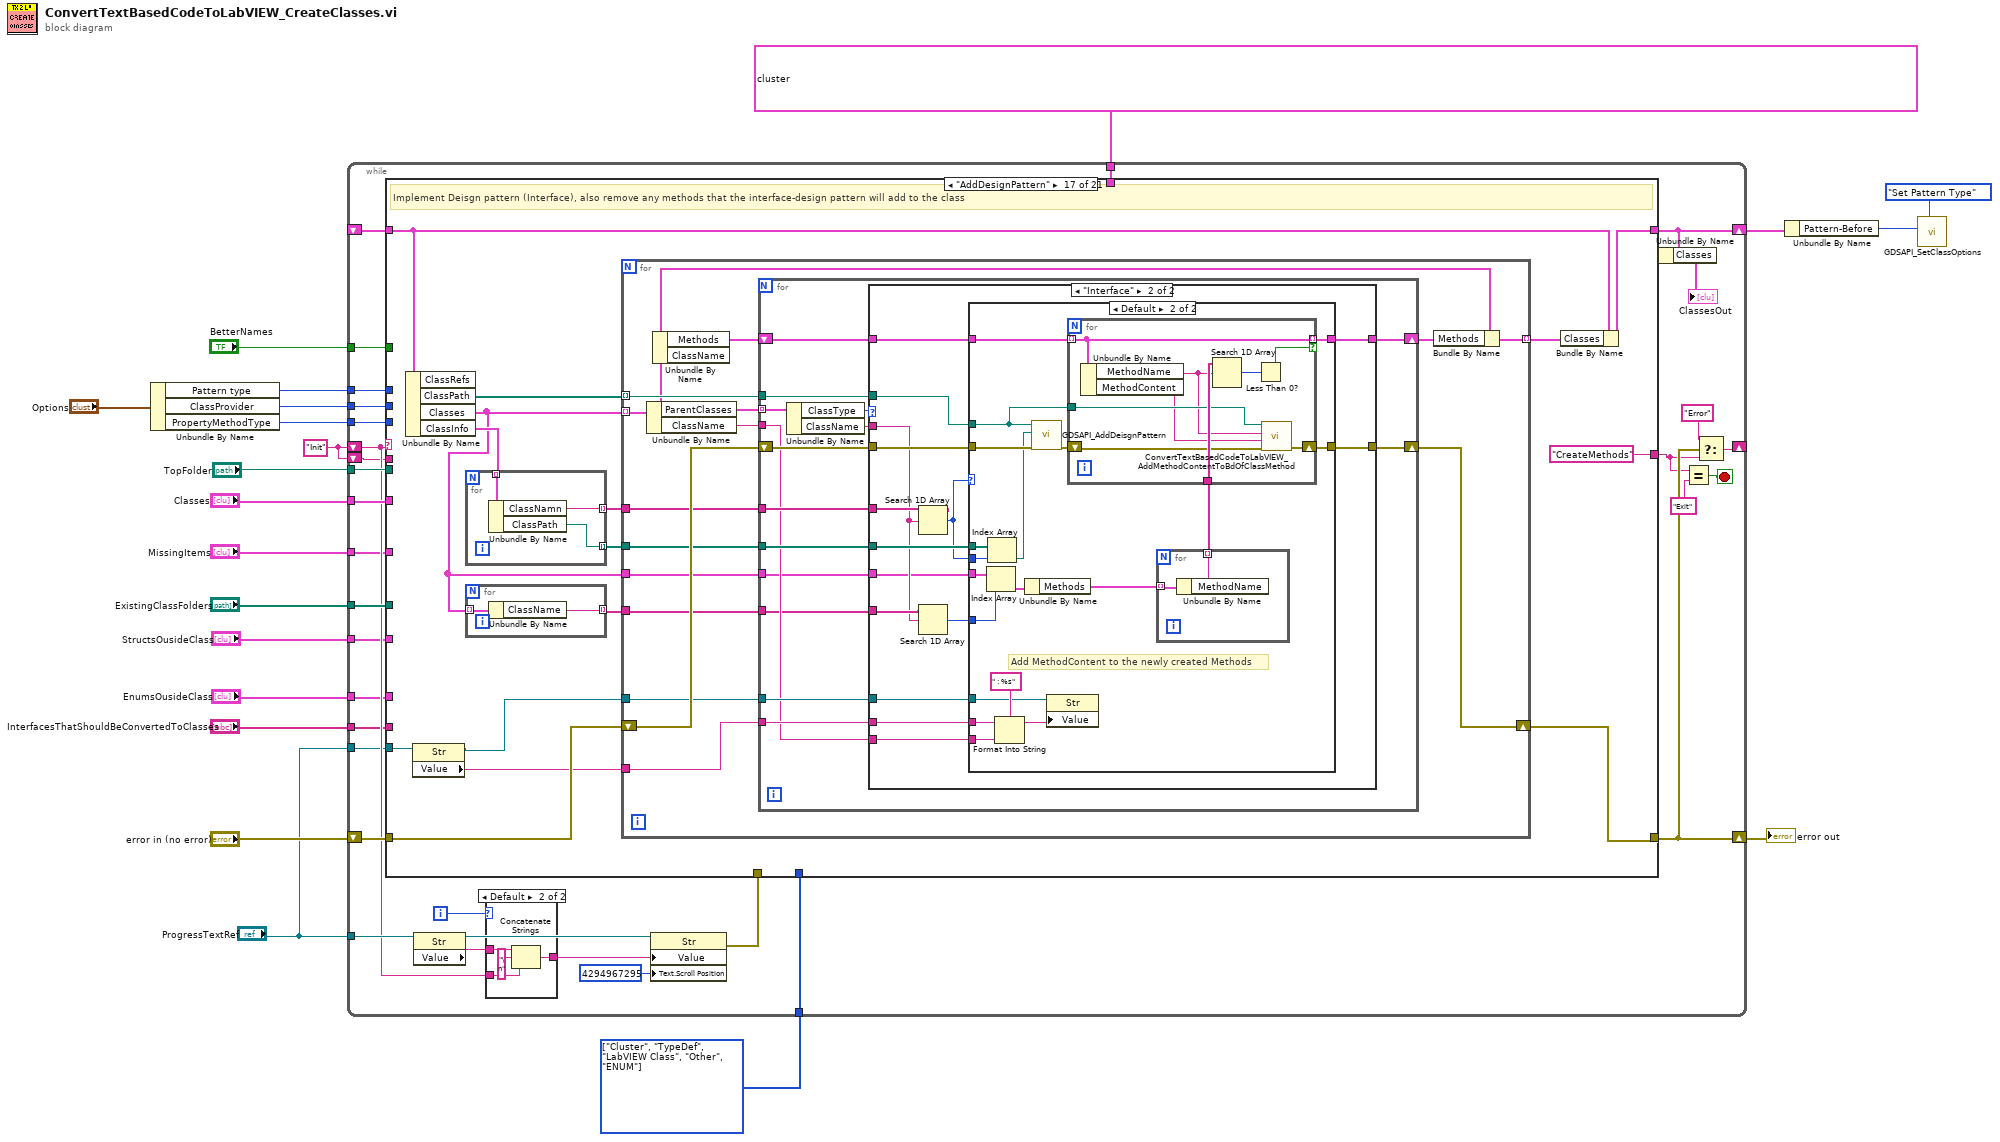
[diagram p0: block diagram]
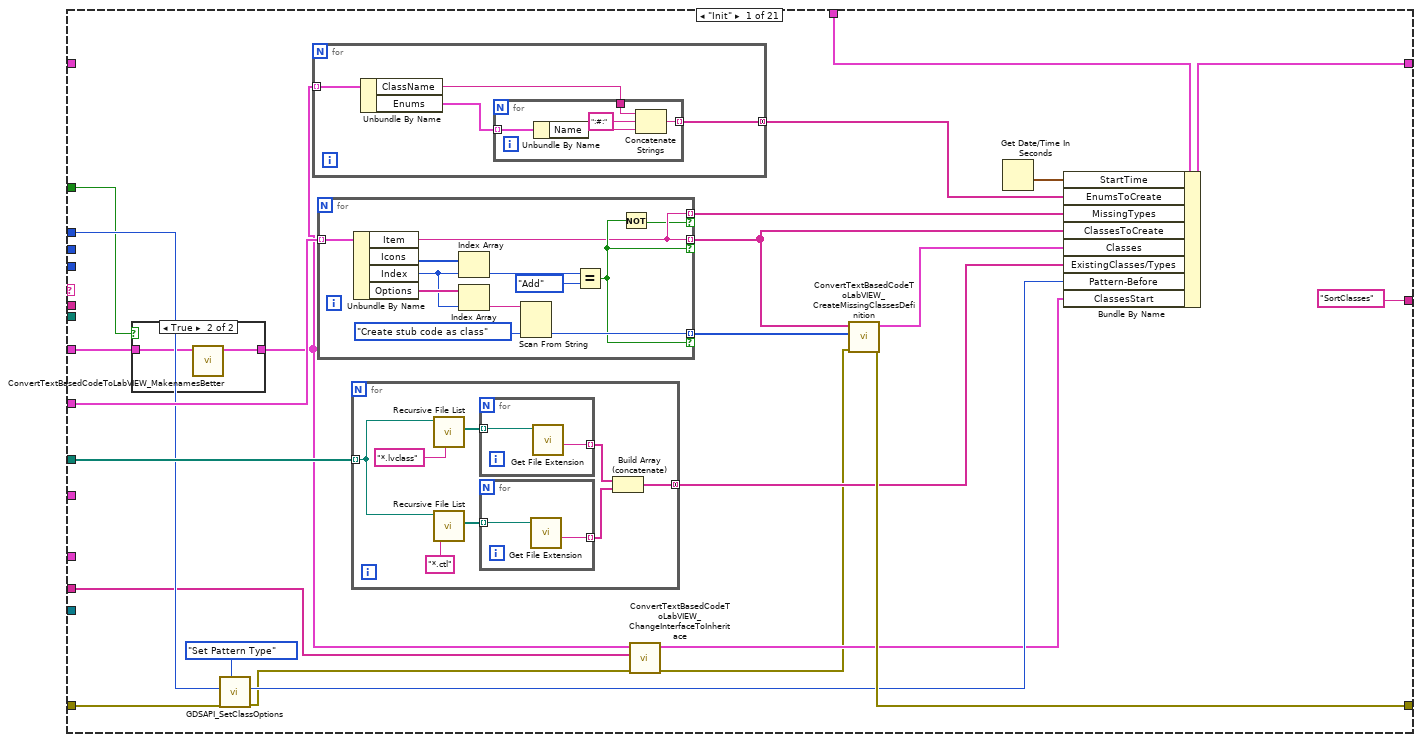
[diagram p3: hidden frame]
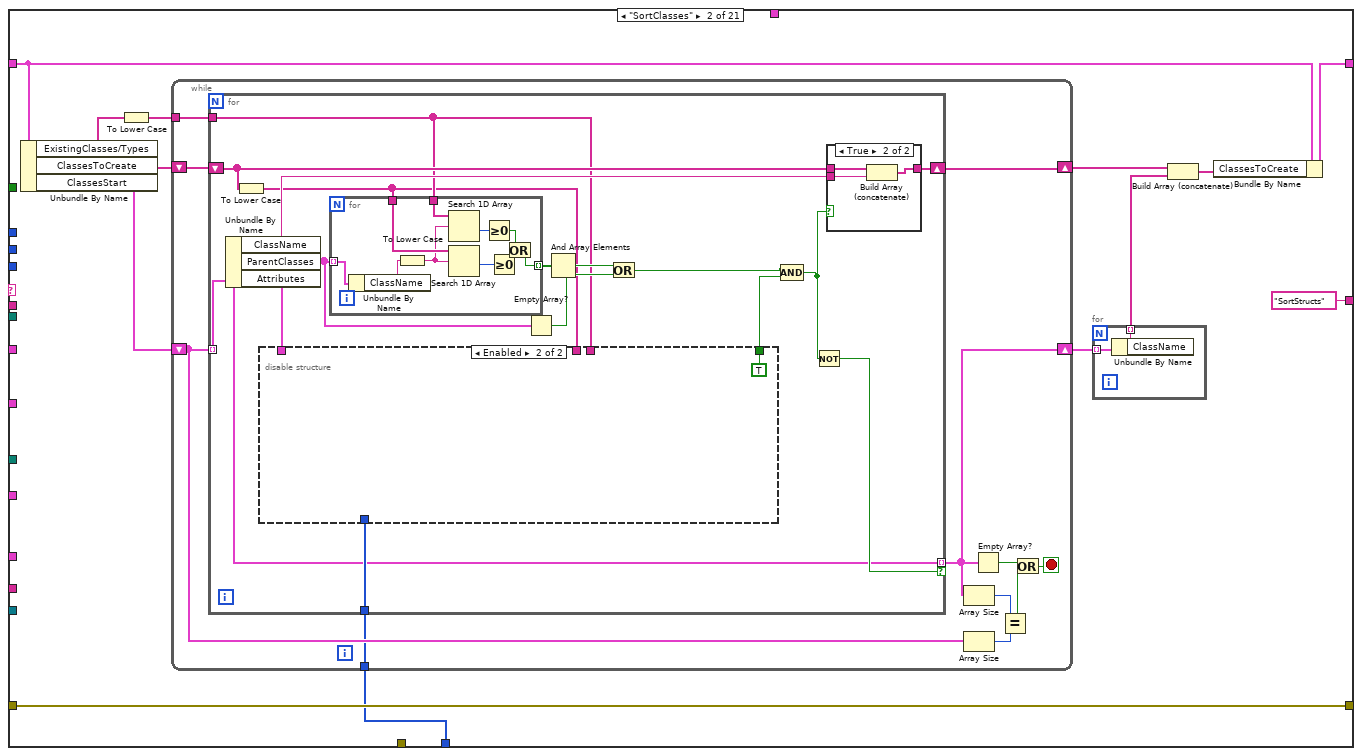
[diagram p5: hidden frame]
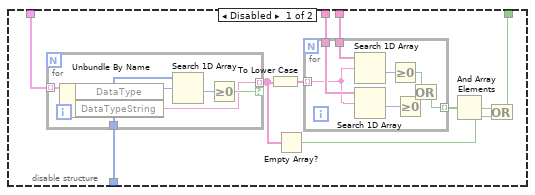
[diagram p6: hidden frame]
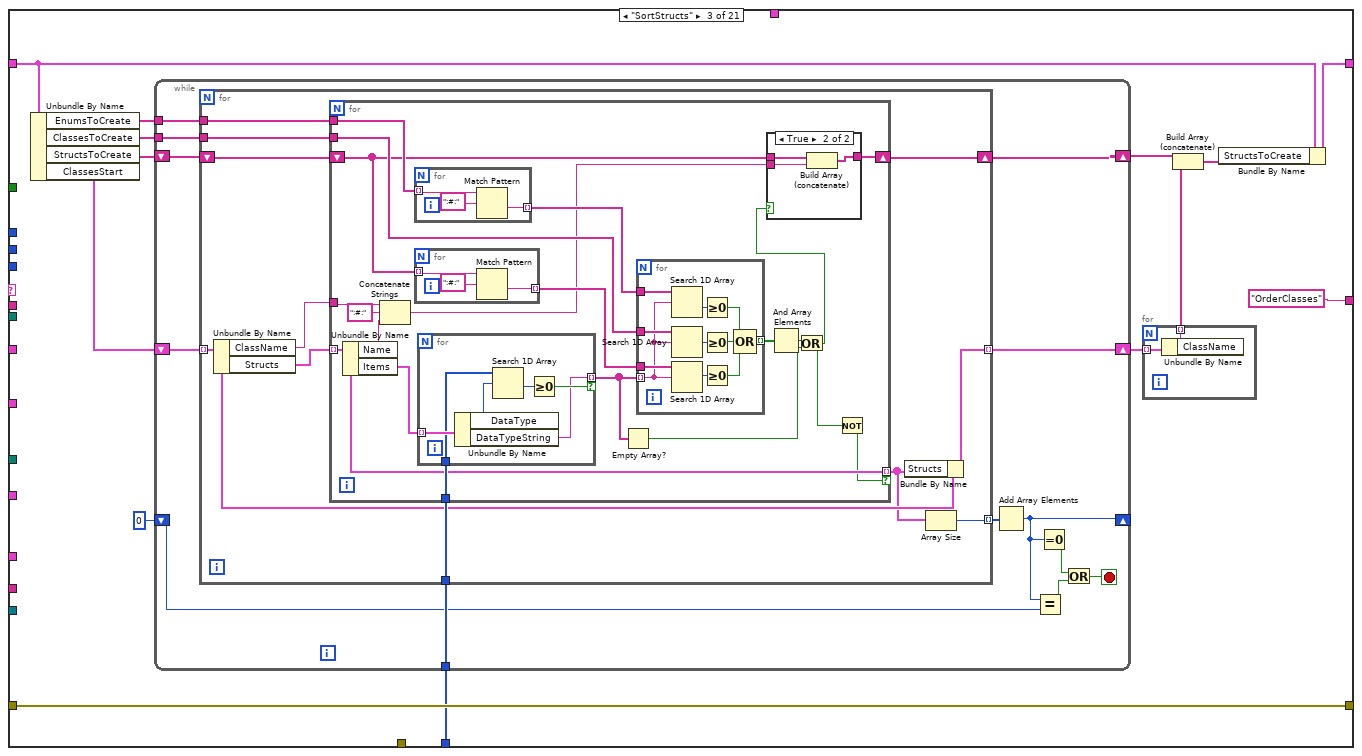
[diagram p8: hidden frame]
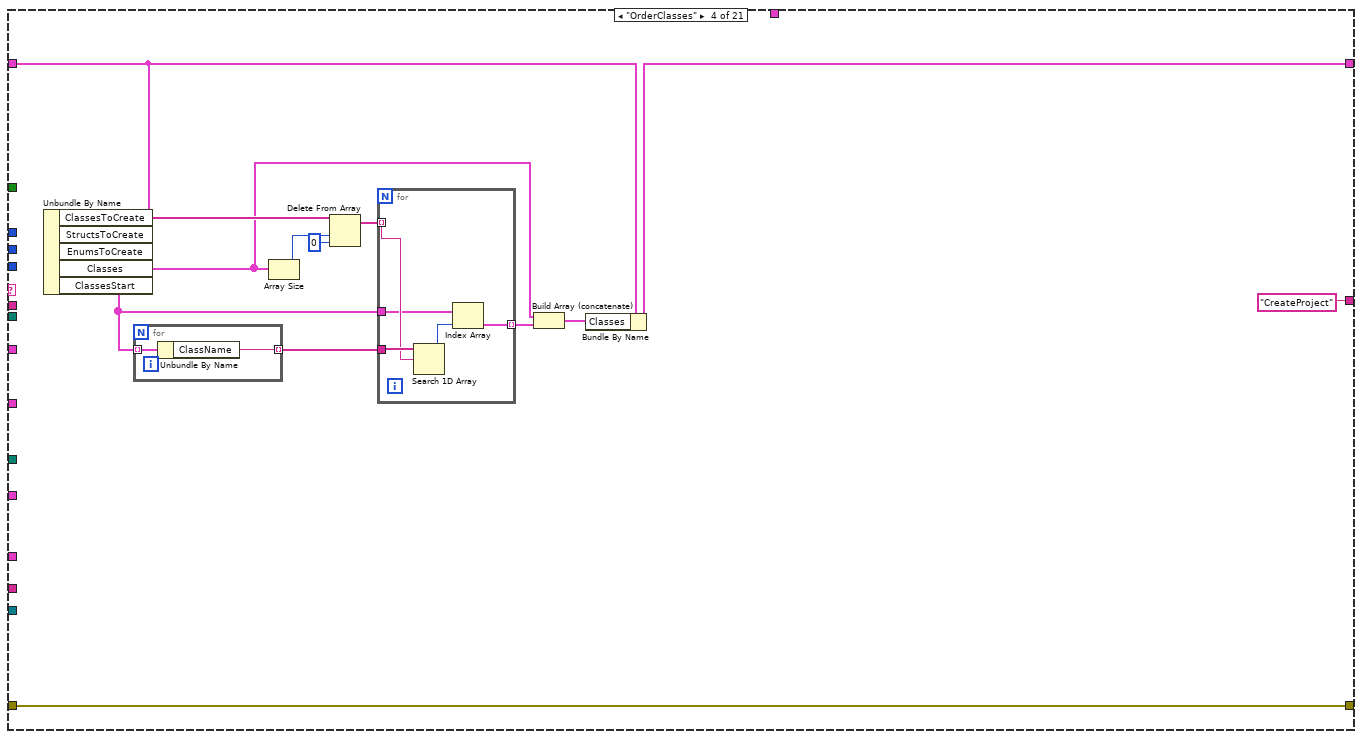
[diagram p10: hidden frame]
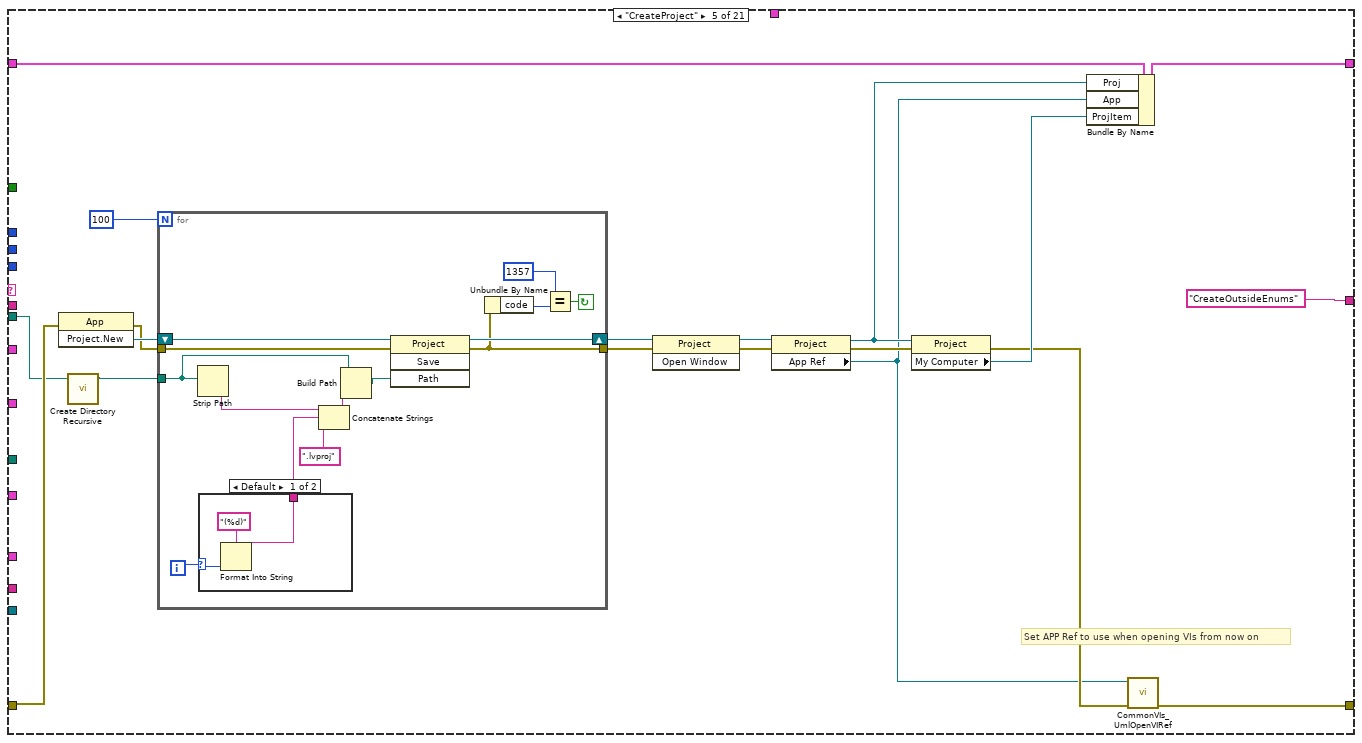
[diagram p11: hidden frame]
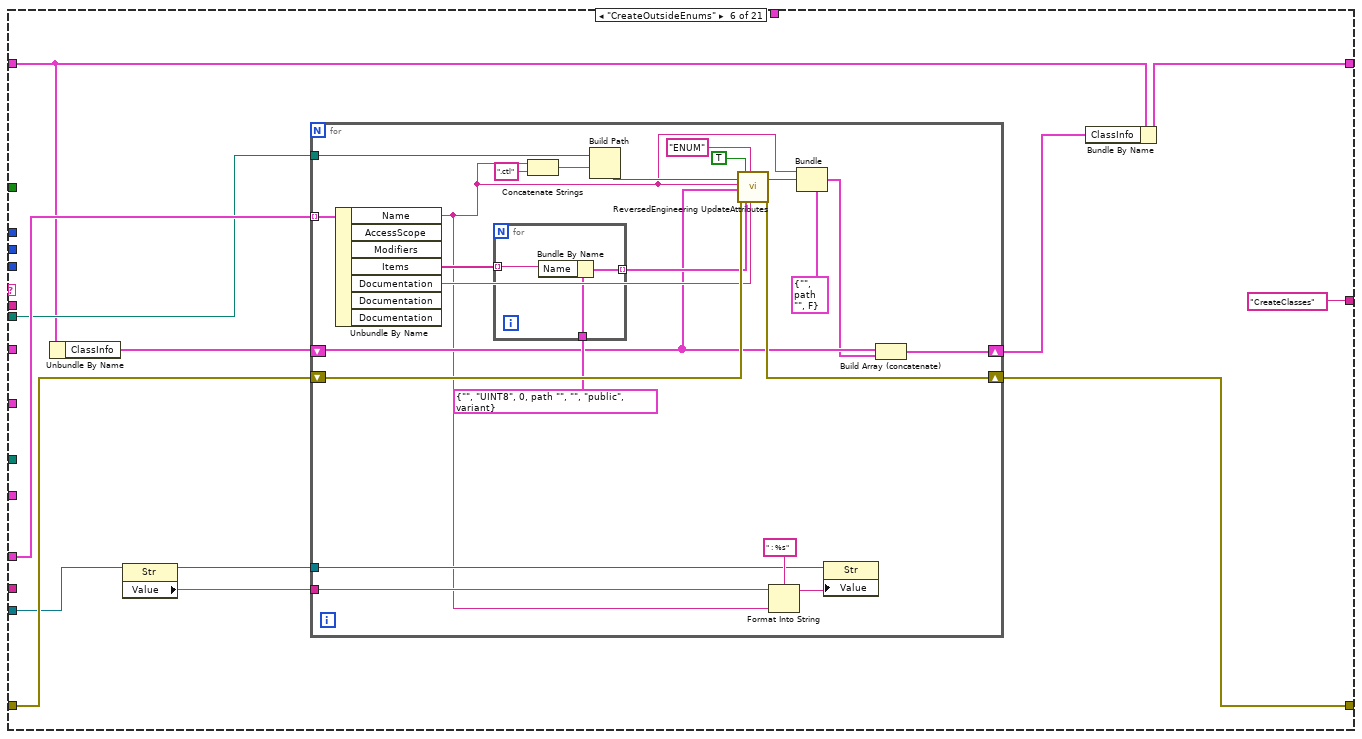
[diagram p13: hidden frame]
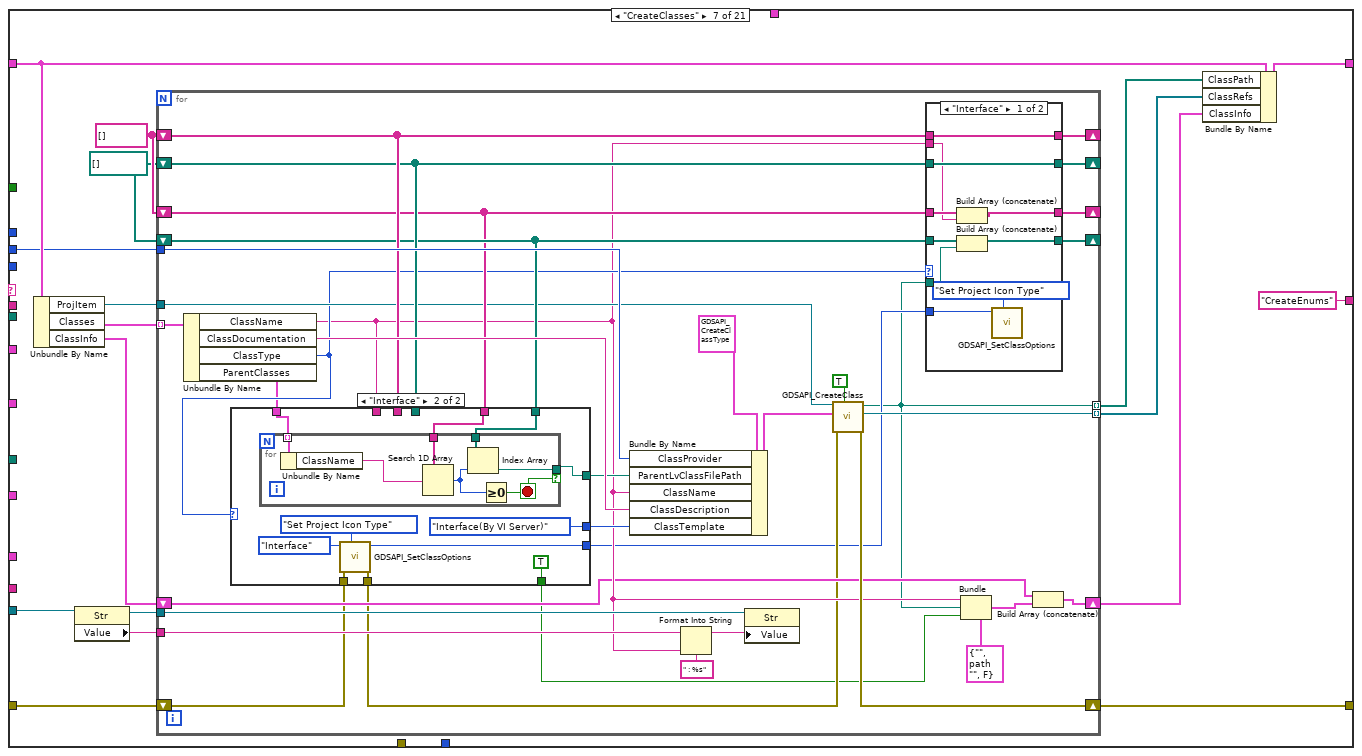
[diagram p14: hidden frame]
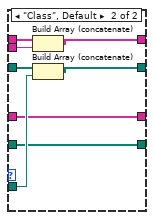
[diagram p15: hidden frame]
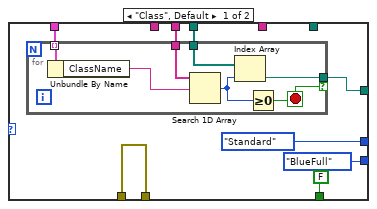
[diagram p16: hidden frame]
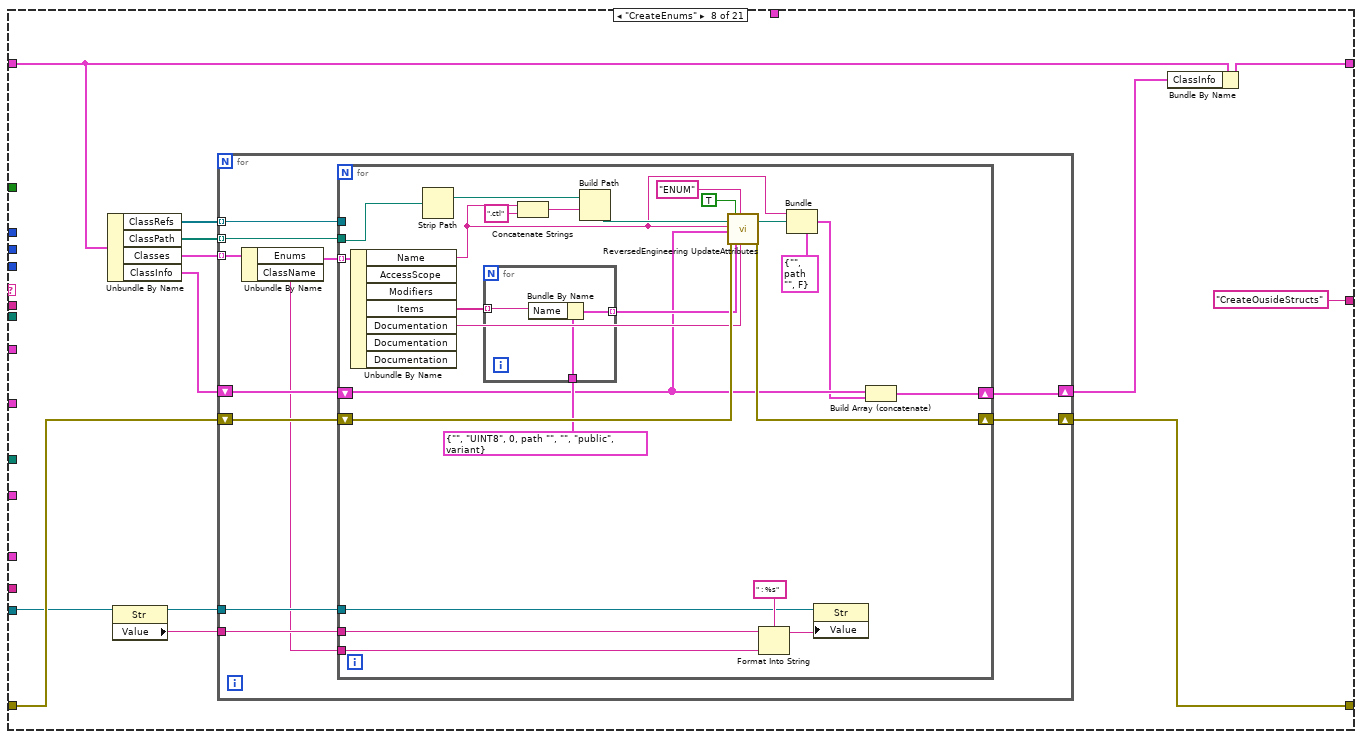
[diagram p17: hidden frame]
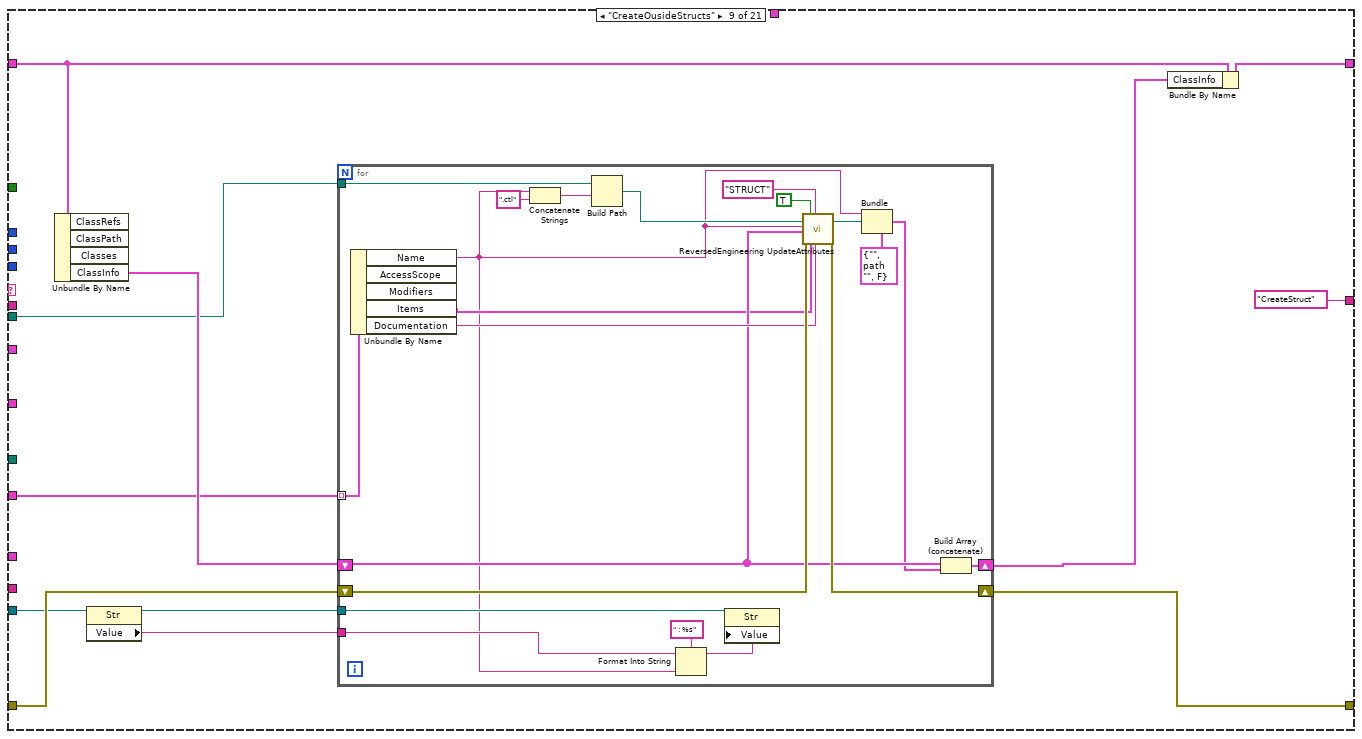
[diagram p18: hidden frame]
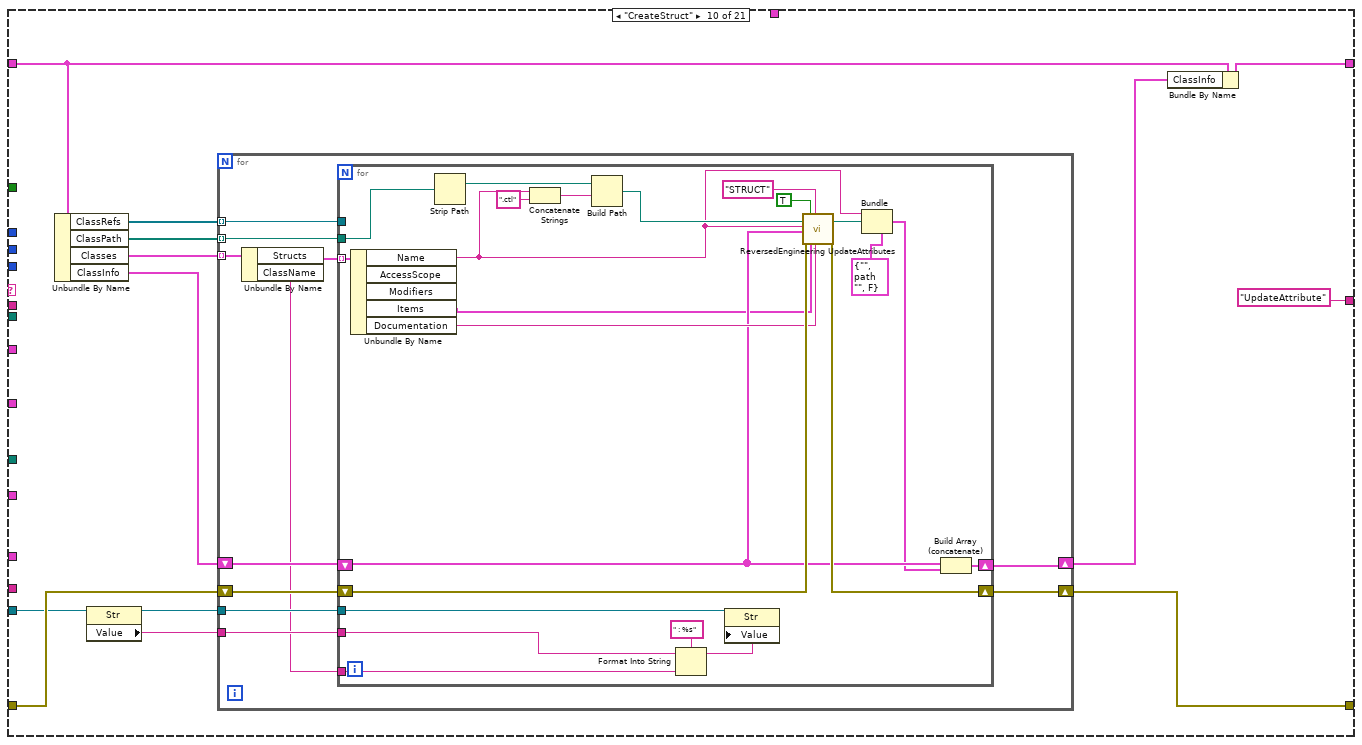
[diagram p19: hidden frame]
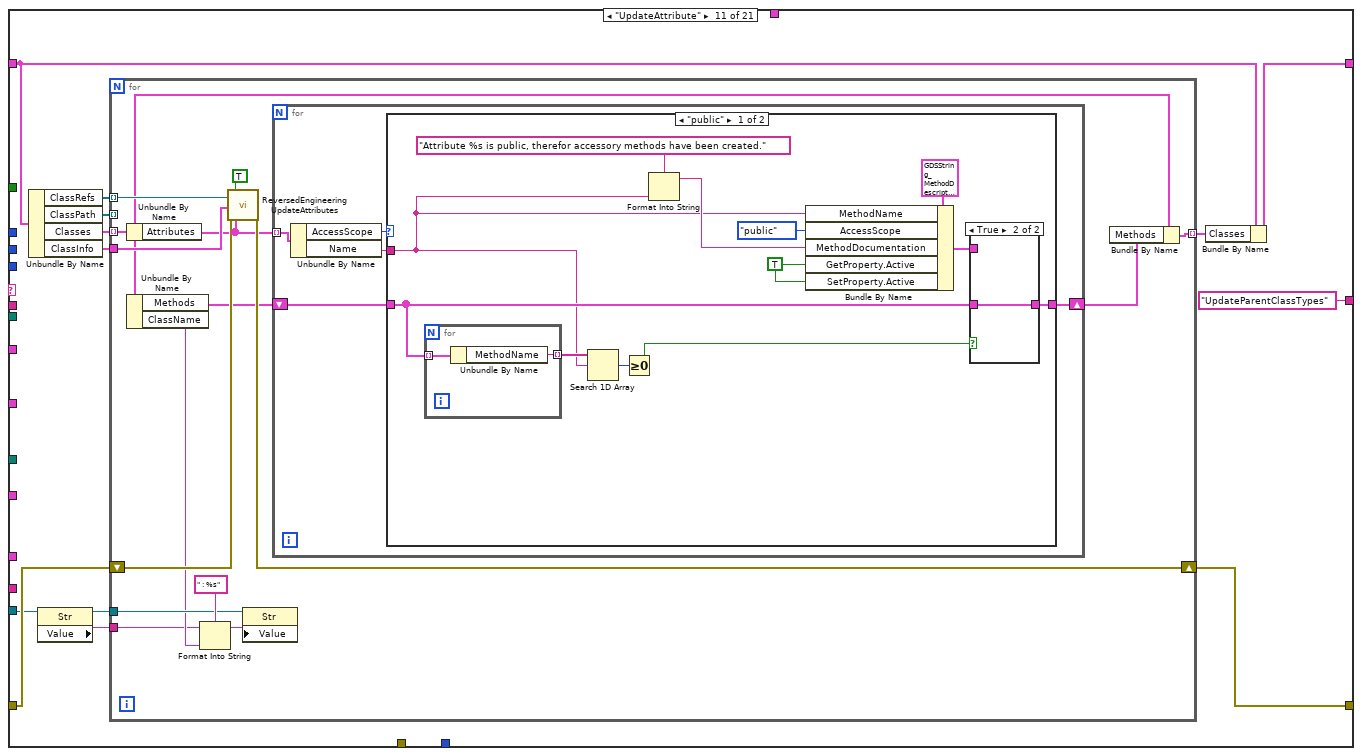
[diagram p20: hidden frame]
diagram:
  w15 = T5[] [enum."Cluster", enum."TypeDef", enum."LabVIEW Class", enum."Other", enum."ENUM"] items=["UINT8", "INT8", "UINT16", "INT16", "UINT32", "INT32", "UINT64", "INT64", "SGL", "DBL", "EXT", "CSG", "CDB", "CXT", "TimeStamp", "STRING", "PATH", "BOOL", "ENUM", "RefNum", "VIRefNum", "LabVIEW Class", "Cluster", "Variant", "TypeDef", "Waveform", "LabVIEW Object", "Other", "void"]
  w10 = "Init"
  n1 = Unbundle By Name("Options") -> ("Pattern type"=w9:T10, "ClassProvider"=w12:T8, "PropertyMethodType"=w11:T9)
  n2 = while {
    shift-right: [w53] -> w20
    shift-left: "error in (no error)" -> [w54]
    shift-right: [w51] -> _
    shift-left: w10 -> [w36]
    tunnel: "TopFolder" -> [w47]
    tunnel: T21 {"App"=refnum, "Proj"=refnum, "ClassesToCreate"=[], "StructsToCreate"=[], "EnumsToCreate"=[], "Classes"=[], "ProjItem"=refnum, "ClassPath"=[], "ExistingClasses/Types"=[], "ClassRefs"=[], "ClassInfo"=[], "StartTime"=timestamp(0 s since 1904-01-01), "MissingTypes"=[], "Pattern-Before"=0, "ClassesStart"=[{"ClassName"="Program", "AccessScope"=enum."public", "Modifiers"=[], "ClassDocumentation"="", "Methods"=[{"ReturnType"={"Name"="", "DataType"=enum."void", "ArrayDim"=0, "CtrlPath"=path "", "DataTypeString"="void", "AccessScope"=enum."public", "InitialData"=variant(string "")}, "MethodName"="Main", "AccessScope"=enum."public", "Modifiers"=[enum."static"], "MethodDocumentation"="", "MethodContent"="public static void Main(string[] args)\n        {\n            // Create a subject and the observable, inject the subject into the observable\n            Subject subject = new Subject();\n            SubjectObservable observable = new SubjectObservable(subject);\n\n            //Create two observers\n            SubjectObserver zeus = new SubjectObserver(observable, \"Zeus\");\n            SubjectObserver ares = new SubjectObserver(observable, \"Ares\");\n            \n            // Run a loop and trigger the observer\n            for (int i = 0; i < 5; i++)\n            {\n                Console.WriteLine(\"Counter: \" + subject.Counter);\n                observable.inspectSubject();\n\n            }\n\n            Console.ReadLine();\n        }", "MethodArguments"=[{"Name"="args", "DataType"=enum."STRING", "ArrayDim"=1, "CtrlPath"=path "", "DataTypeString"="string[]", "AccessScope"=enum."public", "InitialData"=variant(string "")}], "GetProperty"={"Active"=FALSE, "AccessScope"=enum."public", "Code"=""}, "SetProperty"={"Active"=FALSE, "AccessScope"=enum."public", "Code"=""}}], "ParentClasses"=[], "ClassType"=enum."Class", "Owner"="Test", "OwnerType"=enum."Package/NameSpace", "Generics"=[], "Attributes"=[{"Name"="MyUINT8", "DataType"=enum."UINT8", "ArrayDim"=0, "CtrlPath"=path "", "DataTypeString"="", "AccessScope"=enum."public", "InitialData"=variant}], "Enums"=[{"Name"="MyEnum", "AccessScope"=enum."public", "Modifiers"=[], "Items"=["A1", "A2"], "Documentation"="My Enum Doc"}], "Structs"=[{"Name"="MyStruct", "AccessScope"=enum."public", "Modifiers"=[], "Items"=[{"Name"="MyObject", "DataType"=enum."LabVIEW Class", "ArrayDim"=1, "CtrlPath"=path "", "DataTypeString"="Program", "AccessScope"=enum."public", "InitialData"=variant}, {"Name"="Sträng", "DataType"=enum."STRING", "ArrayDim"=0, "CtrlPath"=path "", "DataTypeString"="", "AccessScope"=enum."public", "InitialData"=variant}], "Documentation"="Struct Doc"}]}, {"ClassName"="Subject", "AccessScope"=enum."public", "Modifiers"=[], "ClassDocumentation"="Class Subject - It has a counter object that increases everytime you inspect it", "Methods"=[{"ReturnType"={"Name"="", "DataType"=enum."INT32", "ArrayDim"=0, "CtrlPath"=path "", "DataTypeString"="int", "AccessScope"=enum."public", "InitialData"=variant(string "")}, "MethodName"="Counter", "AccessScope"=enum."public", "Modifiers"=[], "MethodDocumentation"="", "MethodContent"="public int Counter\n        {\n            get\n            {\n                return ++_counter;\n            }\n        }", "MethodArguments"=[], "GetProperty"={"Active"=TRUE, "AccessScope"=enum."public", "Code"="return ++_counter;"}, "SetProperty"={"Active"=FALSE, "AccessScope"=enum."public", "Code"=""}}], "ParentClasses"=[], "ClassType"=enum."Class", "Owner"="Test", "OwnerType"=enum."Package/NameSpace", "Generics"=[], "Attributes"=[{"Name"="_counter", "DataType"=enum."INT32", "ArrayDim"=0, "CtrlPath"=path "", "DataTypeString"="int", "AccessScope"=enum."private", "InitialData"=variant(string "")}], "Enums"=[], "Structs"=[]}, {"ClassName"="SubjectObservable", "AccessScope"=enum."public", "Modifiers"=[], "ClassDocumentation"="Class Subject Observable - The observable object that observes the subject and notifies the observers", "Methods"=[{"ReturnType"={"Name"="", "DataType"=enum."LabVIEW Object", "ArrayDim"=0, "CtrlPath"=path "", "DataTypeString"="SubjectObservable", "AccessScope"=enum."public", "InitialData"=variant(string "")}, "MethodName"="SubjectObservable", "AccessScope"=enum."public", "Modifiers"=[], "MethodDocumentation"="Accept a subject instance which we shall observe", "MethodContent"="public SubjectObservable(Subject subject)\n        {\n            _subjectObservers = new List<IObserver<Subject>>();\n            _subject = subject;\n\n        }", "MethodArguments"=[{"Name"="subject", "DataType"=enum."LabVIEW Object", "ArrayDim"=0, "CtrlPath"=path "", "DataTypeString"="Subject", "AccessScope"=enum."public", "InitialData"=variant(string "")}], "GetProperty"={"Active"=FALSE, "AccessScope"=enum."public", "Code"=""}, "SetProperty"={"Active"=FALSE, "AccessScope"=enum."public", "Code"=""}}, {"ReturnType"={"Name"="", "DataType"=enum."Other", "ArrayDim"=0, "CtrlPath"=path "", "DataTypeString"="IDisposable", "AccessScope"=enum."public", "InitialData"=variant(string "")}, "MethodName"="Subscribe", "AccessScope"=enum."public", "Modifiers"=[], "MethodDocumentation"="This method allows the observers to attach themselves. It returns a disposer object to the observer\nwhich the observer can utilize to unsubscribe", "MethodContent"="public IDisposable Subscribe(IObserver<Subject> observer)\n        {\n            if (!_subjectObservers.Contains(observer))\n            {\n                _subjectObservers.Add(observer);\n            }\n\n            return new Disposer(_subjectObservers, observer);\n        }", "MethodArguments"=[{"Name"="observer", "DataType"=enum."Other", "ArrayDim"=0, "CtrlPath"=path "", "DataTypeString"="IObserver<Subject>", "AccessScope"=enum."public", "InitialData"=variant(string "")}], "GetProperty"={"Active"=FALSE, "AccessScope"=enum."public", "Code"=""}, "SetProperty"={"Active"=FALSE, "AccessScope"=enum."public", "Code"=""}}, {"ReturnType"={"Name"="", "DataType"=enum."void", "ArrayDim"=0, "CtrlPath"=path "", "DataTypeString"="void", "AccessScope"=enum."public", "InitialData"=variant(string "")}, "MethodName"="inspectSubject", "AccessScope"=enum."public", "Modifiers"=[enum."event"], "MethodDocumentation"="This method is used to inspect the subject over time. Usually used with a timer or an event", "MethodContent"="event\n        public void inspectSubject()\n        {\n            foreach (IObserver<Subject> observer in _subjectObservers)\n            {\n                observer.OnNext(_subject);\n            }\n        }", "MethodArguments"=[], "GetProperty"={"Active"=FALSE, "AccessScope"=enum."public", "Code"=""}, "SetProperty"={"Active"=FALSE, "AccessScope"=enum."public", "Code"=""}}], "ParentClasses"=[{"ClassName"="IObservable", "ClassType"=enum."Undefined"}], "ClassType"=enum."Class", "Owner"="Test", "OwnerType"=enum."Package/NameSpace", "Generics"=["Subject"], "Attributes"=[{"Name"="_subjectObservers", "DataType"=enum."Other", "ArrayDim"=1, "CtrlPath"=path "", "DataTypeString"="IObserver<Subject>", "AccessScope"=enum."private", "InitialData"=variant(string "")}, {"Name"="_subject", "DataType"=enum."LabVIEW Object", "ArrayDim"=0, "CtrlPath"=path "", "DataTypeString"="Subject", "AccessScope"=enum."private", "InitialData"=variant(string "")}], "Enums"=[], "Structs"=[]}, {"ClassName"="SubjectObserver", "AccessScope"=enum."public", "Modifiers"=[], "ClassDocumentation"="Class Subject Observer - The object that attaches itself to a observable and recieves notifications", "Methods"=[{"ReturnType"={"Name"="", "DataType"=enum."LabVIEW Object", "ArrayDim"=0, "CtrlPath"=path "", "DataTypeString"="SubjectObserver", "AccessScope"=enum."public", "InitialData"=variant(string "")}, "MethodName"="SubjectObserver", "AccessScope"=enum."public", "Modifiers"=[], "MethodDocumentation"="", "MethodContent"="public SubjectObserver(IObservable<Subject> provider, string instanceName)\n        {\n            if (provider != null)\n            {\n                _disposer = provider.Subscribe(this);\n                _instaceName = instanceName;\n            }\n        }", "MethodArguments"=[{"Name"="provider", "DataType"=enum."Other", "ArrayDim"=0, "CtrlPath"=path "", "DataTypeString"="IObservable<Subject>", "AccessScope"=enum."public", "InitialData"=variant(string "")}, {"Name"="instanceName", "DataType"=enum."STRING", "ArrayDim"=0, "CtrlPath"=path "", "DataTypeString"="string", "AccessScope"=enum."public", "InitialData"=variant(string "")}], "GetProperty"={"Active"=FALSE, "AccessScope"=enum."public", "Code"=""}, "SetProperty"={"Active"=FALSE, "AccessScope"=enum."public", "Code"=""}}, {"ReturnType"={"Name"="", "DataType"=enum."void", "ArrayDim"=0, "CtrlPath"=path "", "DataTypeString"="void", "AccessScope"=enum."public", "InitialData"=variant(string "")}, "MethodName"="OnNext", "AccessScope"=enum."public", "Modifiers"=[], "MethodDocumentation"="The observable invokes this method to pass the Subject object to the observer", "MethodContent"="public void OnNext(Subject value)\n        {\n            Console.WriteLine(\"[\" + _instaceName + \"] \" + value.Counter);\n        }", "MethodArguments"=[{"Name"="value", "DataType"=enum."LabVIEW Object", "ArrayDim"=0, "CtrlPath"=path "", "DataTypeString"="Subject", "AccessScope"=enum."public", "InitialData"=variant(string "")}], "GetProperty"={"Active"=FALSE, "AccessScope"=enum."public", "Code"=""}, "SetProperty"={"Active"=FALSE, "AccessScope"=enum."public", "Code"=""}}, {"ReturnType"={"Name"="", "DataType"=enum."void", "ArrayDim"=0, "CtrlPath"=path "", "DataTypeString"="void", "AccessScope"=enum."public", "InitialData"=variant(string "")}, "MethodName"="OnCompleted", "AccessScope"=enum."public", "Modifiers"=[], "MethodDocumentation"="Usually called when a transmission is complete. Not implemented.", "MethodContent"="public void OnCompleted()\n        {\n            throw new NotImplementedException();\n        }", "MethodArguments"=[], "GetProperty"={"Active"=FALSE, "AccessScope"=enum."public", "Code"=""}, "SetProperty"={"Active"=FALSE, "AccessScope"=enum."public", "Code"=""}}, {"ReturnType"={"Name"="", "DataType"=enum."void", "ArrayDim"=0, "CtrlPath"=path "", "DataTypeString"="void", "AccessScope"=enum."public", "InitialData"=variant(string "")}, "MethodName"="OnError", "AccessScope"=enum."public", "Modifiers"=[], "MethodDocumentation"="Usually called when there was an error. Didn't implement.", "MethodContent"="public void OnError(Exception error)\n        {\n            throw new NotImplementedException();\n        }", "MethodArguments"=[{"Name"="error", "DataType"=enum."Other", "ArrayDim"=0, "CtrlPath"=path "", "DataTypeString"="Exception", "AccessScope"=enum."public", "InitialData"=variant(string "")}], "GetProperty"={"Active"=FALSE, "AccessScope"=enum."public", "Code"=""}, "SetProperty"={"Active"=FALSE, "AccessScope"=enum."public", "Code"=""}}, {"ReturnType"={"Name"="", "DataType"=enum."void", "ArrayDim"=0, "CtrlPath"=path "", "DataTypeString"="void", "AccessScope"=enum."public", "InitialData"=variant(string "")}, "MethodName"="Dispose", "AccessScope"=enum."public", "Modifiers"=[], "MethodDocumentation"="Invoke the disposer recieved from the observable. This will unsubscribe", "MethodContent"="public void Dispose()\n        {\n            _disposer.Dispose();\n        }", "MethodArguments"=[], "GetProperty"={"Active"=FALSE, "AccessScope"=enum."public", "Code"=""}, "SetProperty"={"Active"=FALSE, "AccessScope"=enum."public", "Code"=""}}], "ParentClasses"=[{"ClassName"="IObserver", "ClassType"=enum."Undefined"}], "ClassType"=enum."Class", "Owner"="Test", "OwnerType"=enum."Package/NameSpace", "Generics"=["Subject"], "Attributes"=[{"Name"="_disposer", "DataType"=enum."Other", "ArrayDim"=0, "CtrlPath"=path "", "DataTypeString"="IDisposable", "AccessScope"=enum."private", "InitialData"=variant(string "")}, {"Name"="_instaceName", "DataType"=enum."STRING", "ArrayDim"=0, "CtrlPath"=path "", "DataTypeString"="string", "AccessScope"=enum."private", "InitialData"=variant(string "")}], "Enums"=[], "Structs"=[]}, {"ClassName"="Disposer", "AccessScope"=enum."private", "Modifiers"=[], "ClassDocumentation"="Private class Disposer: Implements the IDisposable. Observable returns an instance to the observer for easy unsubscription\nprivate", "Methods"=[{"ReturnType"={"Name"="", "DataType"=enum."LabVIEW Object", "ArrayDim"=0, "CtrlPath"=path "", "DataTypeString"="Disposer", "AccessScope"=enum."public", "InitialData"=variant(string "")}, "MethodName"="Disposer", "AccessScope"=enum."public", "Modifiers"=[], "MethodDocumentation"="", "MethodContent"="public Disposer(List<IObserver<Subject>> _subObservers, IObserver<Subject> observer)\n            {\n                _subjectObservers = _subObservers;\n                _observer = observer;\n            }", "MethodArguments"=[{"Name"="_subObservers", "DataType"=enum."Other", "ArrayDim"=1, "CtrlPath"=path "", "DataTypeString"="IObserver<Subject>", "AccessScope"=enum."public", "InitialData"=variant(string "")}, {"Name"="observer", "DataType"=enum."Other", "ArrayDim"=0, "CtrlPath"=path "", "DataTypeString"="IObserver<Subject>", "AccessScope"=enum."public", "InitialData"=variant(string "")}], "GetProperty"={"Active"=FALSE, "AccessScope"=enum."public", "Code"=""}, "SetProperty"={"Active"=FALSE, "AccessScope"=enum."public", "Code"=""}}, {"ReturnType"={"Name"="", "DataType"=enum."void", "ArrayDim"=0, "CtrlPath"=path "", "DataTypeString"="void", "AccessScope"=enum."public", "InitialData"=variant(string "")}, "MethodName"="Dispose", "AccessScope"=enum."public", "Modifiers"=[], "MethodDocumentation"="", "MethodContent"="public void Dispose()\n            {\n                if (_subjectObservers.Contains(_observer))\n                {\n                    _subjectObservers.Remove(_observer);\n                }\n            }", "MethodArguments"=[], "GetProperty"={"Active"=FALSE, "AccessScope"=enum."public", "Code"=""}, "SetProperty"={"Active"=FALSE, "AccessScope"=enum."public", "Code"=""}}], "ParentClasses"=[{"ClassName"="IDisposable", "ClassType"=enum."Undefined"}], "ClassType"=enum."Class", "Owner"="SubjectObservable", "OwnerType"=enum."Class", "Generics"=[], "Attributes"=[{"Name"="_subjectObservers", "DataType"=enum."Other", "ArrayDim"=1, "CtrlPath"=path "", "DataTypeString"="IObserver<Subject>", "AccessScope"=enum."private", "InitialData"=variant(string "")}, {"Name"="_observer", "DataType"=enum."Other", "ArrayDim"=0, "CtrlPath"=path "", "DataTypeString"="IObserver<Subject>", "AccessScope"=enum."private", "InitialData"=variant(string "")}], "Enums"=[], "Structs"=[]}]} -> [w46]
    shift-right: [w31] -> w6
    shift-left: _ -> [w45]
    tunnel: "Classes" -> [w44]
    tunnel: "MissingItems" -> [w28]
    tunnel: w15 -> [w43]
    tunnel: w12 -> [w42]
    tunnel: "ExistingClassFolders" -> [w41]
    tunnel: "ProgressTextRef" -> [w40]
    tunnel: "ProgressTextRef" -> [w32]
    tunnel: w11 -> [w30]
    shift-left: w10 -> [w29]
    tunnel: w9 -> [w27]
    tunnel: "EnumsOusideClass" -> [w25]
    tunnel: "StructsOusideClass" -> [w24]
    tunnel: "InterfacesThatShouldBeConvertedToClasses" -> [w23]
    tunnel: "BetterNames" -> [w22]
    i -> [w38]
    stop <- w48 stop-if-true
    n3 = property class="Str"(reference=w40) -> (reference out=w39:refnum<vi>, "Value"=w35:string)  [unwired: 1 in, 1 out]
    n4 = case shown="Default" w38 {
      tunnel: [w55 w57] -> w37
      tunnel: w36 -> [w55 w58]
      tunnel: w35 -> [_ w59]
      frame 0 {
      }
      frame Default {
        n5 = Concatenate Strings(w59, "\n" ("string"), w58) -> (w57:string)
      }
    }
    n6 = property class="Str"(reference=w39, "Value"=w37, "Text.Scroll Position"=u32 4294967295) -> (error out=w33:errorcluster)  [unwired: 1 in, 1 out]
    n7 = case shown="\"AddDesignPattern\"" w36 {
      tunnel: w54 -> [w70 w131 w214 w299 w324 w350 w391 w488 w543 w574 w623 w670 w704 w735 w790 w855 w887 w979 w1010 w1039 w1050]
      tunnel: [w75 w131 w214 w299 w315 w349 w390 w487 w542 w573 w622 w670 w704 w734 w789 w854 w879 w978 w1010 w1038 w1049] -> w53
      tunnel: ["SortClasses" "SortStructs" "OrderClasses" "CreateProject" "CreateOutsideEnums" "CreateClasses" "CreateEnums" "CreateOusideStructs" "CreateStruct" "UpdateAttribute" "UpdateParentClassTypes" "UpdateMethodTypes" "UpdateConstructors" "UpdateDestructors" "AddInterfaceMethods" "AddDesignPattern" "CreateMethods" "SaveAll" "Done" "CloseDown" "Exit"] -> w50
      tunnel: w47 -> [_ _ _ _ w308 w346 _ _ w536 _ _ _ _ _ _ _ _ _ _ _ _]
      tunnel: w46 -> [w83 _ _ _ _ _ _ _ _ _ _ _ _ _ _ _ _ _ _ _ _]
      tunnel: [w82 w128 w211 w289 w320 w343 w388 w490 w545 w576 w617 w671 w705 w739 w794 w853 w877 w977 w1009 w1047 w1052] -> w31
      tunnel: w45 -> [_ w130 w213 w297 w321 w344 w396 w495 w547 w581 w624 w669 w703 w738 w793 w853 w878 w977 w1009 w1047 w1052]
      tunnel: w44 -> [w62 _ _ _ _ _ _ _ _ _ _ _ _ _ _ _ _ _ _ _ _]
      tunnel: w28 -> [w81 _ _ _ _ _ _ _ _ _ _ _ _ _ _ _ _ _ _ _ _]
      tunnel: w43 -> [_ w125 w210 _ _ _ _ _ _ _ _ _ _ _ _ _ _ _ _ _ _]
      tunnel: w42 -> [_ _ _ _ _ _ w394 _ _ _ _ _ _ _ _ _ _ _ _ _ _]
      tunnel: w41 -> [w74 _ _ _ _ _ _ _ _ _ _ _ _ _ _ _ _ _ _ _ _]
      tunnel: w33 -> [_ _ _ _ _ _ _ _ _ _ _ _ _ _ _ _ _ _ _ _ _]
      tunnel: w32 -> [_ _ _ _ _ w348 w384 w486 w541 w571 w620 _ _ _ _ w852 w882 w976 _ w1028 _]
      tunnel: w30 -> [_ _ _ _ _ _ _ _ _ _ _ _ _ _ _ _ _ w973 _ _ _]
      tunnel: w29 -> [_ _ _ _ _ _ _ _ _ _ _ _ _ _ _ _ _ _ _ _ _]
      tunnel: w27 -> [w69 _ _ _ _ _ _ _ _ _ _ _ _ _ _ _ _ _ _ _ _]
      tunnel: w25 -> [_ _ _ _ _ w347 _ _ _ _ _ _ _ _ _ _ _ _ _ _ _]
      tunnel: w24 -> [_ _ _ _ _ _ _ _ w537 _ _ _ _ _ _ _ _ _ _ _ _]
      tunnel: w23 -> [w66 _ _ _ _ _ _ _ _ _ _ _ _ _ _ _ _ _ _ _ _]
      tunnel: w22 -> [w60 _ _ _ _ _ _ _ _ _ _ _ _ _ _ _ _ _ _ _ _]
      frame "Init" {
        n8 = case shown="True" w60 {
          tunnel: w62 -> [w84 w86]
          tunnel: [w84 w85] -> w61
          frame False {
          }
          frame True {
            n9 = call <resource>:"ConvertTextBasedCodeToLabVIEW_MakenamesBetter.vi"("ClassesIn"=w86) -> ("ClassesOut"=w85:T11[])  [unwired: 10 in]
          }
        }
        n10 = call <resource>:"GDSAPI_SetClassOptions.vi"("SetAction(Set All)"=GDSAPI_SetClassOptionsAction."Set Pattern Type", "error in (no error)"=w70, "PatternIn"=w69) -> ("error out"=w64:errorcluster, "Pattern-Before"=w67:T10)  [unwired: 5 in, 2 out]
        n11 = for {
          tunnel: w61 -> [w102] mode=indexing
          tunnel: [w99] -> w80 mode=concatenating
          n12 = Unbundle By Name(w102) -> ("ClassName"=w100:string, "Enums"=w101:T6[])
          n13 = for {
            tunnel: w101 -> [w107] mode=indexing
            tunnel: w100 -> [w104]
            tunnel: [w103] -> w99 mode=indexing
            n14 = Unbundle By Name(w107) -> ("Name"=w105:string)
            n15 = Concatenate Strings(w104, ":#:" ("string"), w105) -> (w103:string)
          }
        }
        n16 = for {
          tunnel: w81 -> [w119] mode=indexing
          tunnel: [w109] -> w78 mode=indexing if=w110
          tunnel: [w111] -> w77 mode=indexing if=w110
          tunnel: [w109] -> w71 mode=indexing if=w108
          n17 = Unbundle By Name(w119) -> ("Item"=w109:string, "Icons"=w118:T18[], "Index"=w114:i32, "Options"=w115:string[])
          n18 = Index Array(array=w118, index=w114) -> (element=w117:T18)
          n19 = Index Array(array=w115, index=w114) -> (element=w113:string)
          n20 = Scan From String(input string=w113, default 1=ConvertTextBasedCodeToLabVIEW_MissingTypeOptions."Create stub code as class") -> (output 1=w111:T22)  [unwired: 3 in, 3 out]
          n21 = Equal?(x=w117, y=ConvertTextBasedCodeToLabVIEW_MissingTypeIconType."Add") -> (x = y?=w110:bool)
          n22 = Not(x=w110) -> (.not. x?=w108:bool)
        }
        n23 = for {
          tunnel: w74 -> [w88] mode=indexing
          tunnel: [w87] -> w73 mode=concatenating
          n24 = call <vilib>:"Recursive File List.vi"("pattern"="*.lvclass", "Folder Path"=w88) -> ("All Files in Dir"=w92:path[])  [unwired: 5 in, 4 out]
          n25 = call <vilib>:"Recursive File List.vi"("pattern"="*.ctl", "Folder Path"=w88) -> ("All Files in Dir"=w91:path[])  [unwired: 5 in, 4 out]
          n26 = for {
            tunnel: w92 -> [w98] mode=indexing
            tunnel: [w97] -> w90 mode=indexing
            n27 = call <vilib>:"Get File Extension.vi"("file"=w98) -> ("filename without extension"=w97:string)  [unwired: 6 in, 4 out]
          }
          n28 = for {
            tunnel: w91 -> [w96] mode=indexing
            tunnel: [w95] -> w89 mode=indexing
            n29 = call <vilib>:"Get File Extension.vi"("file"=w96) -> ("filename without extension"=w95:string)  [unwired: 6 in, 4 out]
          }
          n30 = Build Array (concatenate)(w90, w89) -> (w87:string[])
        }
        n31 = call <resource>:"ConvertTextBasedCodeToLabVIEW_ChangeInterfaceToInheritace.vi"("error in (no error)"=w64, "InterfacesThatShouldBeConvertedToClasses"=w66, "ClassesIn"=w61) -> ("error out"=w63:errorcluster, "ClassesOut"=w65:T11[])  [unwired: 7 in]
        n32 = call <resource>:"ConvertTextBasedCodeToLabVIEW_CreateMissingClassesDefinition.vi"("error in (no error)"=w63, "Action"=w77, "ClassName"=w78) -> ("error out"=w75:errorcluster, "Classes"=w76:T11[])  [unwired: 7 in]
        n33 = Get Date/Time In Seconds() -> (seconds since 1Jan1904=w72:timestamp)
        n34 = Bundle By Name(cluster=w83, "StartTime"=w72, "EnumsToCreate"=w80, "MissingTypes"=w71, "ClassesToCreate"=w78, "Classes"=w76, "ExistingClasses/Types"=w73, "Pattern-Before"=w67, "ClassesStart"=w65) -> (w82:T21)
      }
      frame "SortClasses" {
        n35 = Unbundle By Name(w130) -> ("ExistingClasses/Types"=w127:string[], "ClassesToCreate"=w129:string[], "ClassesStart"=w120:T11[])
        n36 = To Lower Case(string=w127) -> (all lower case string=w126:string[])
        n37 = while {
          shift-right: [w144] -> w124
          shift-left: w129 -> [w145]
          shift-right: [w142] -> w122
          shift-left: w120 -> [w141]
          tunnel: w126 -> [w136]
          tunnel: w125 -> [w135]
          stop <- w137 stop-if-true
          n38 = for {
            tunnel: w141 -> [w146] mode=indexing
            shift-right: [w156] -> w144
            shift-left: w145 -> [w154]
            tunnel: [w146] -> w142 mode=indexing if=w155
            tunnel: w136 -> [w151]
            tunnel: w135 -> [w153]
            n39 = Unbundle By Name(w146) -> ("ClassName"=w157:string, "ParentClasses"=w160:T14[], "Attributes"=w152:T4[])
            n40 = To Lower Case(string=w154) -> (all lower case string=w150:string[])
            n41 = disable-structure shown="Enabled" {
              disable-tunnel: w153 -> [w171 _]
              disable-tunnel: w152 -> [w169 _]
              disable-tunnel: w151 -> [w168 _]
              disable-tunnel: w150 -> [w167 _]
              disable-tunnel: [w162 TRUE] -> w148
              frame Disabled {
                n42 = for {
                  tunnel: w169 -> [w184] mode=indexing
                  tunnel: w171 -> [w183]
                  tunnel: [w180] -> w163 mode=indexing if=w181
                  n43 = Unbundle By Name(w184) -> ("DataType"=w182:T5, "DataTypeString"=w180:string)
                  n44 = Search 1D Array(1D array=w183, element=w182) -> (index of element=w185:i32)  [unwired: 1 in]
                  n45 = Greater Or Equal To 0?(x=w185) -> (x >= 0?=w181:bool)
                }
                n46 = To Lower Case(string=w163) -> (all lower case string=w166:string[])
                n47 = Empty Array?(array=w163) -> (empty?=w165:bool)
                n48 = for {
                  tunnel: w167 -> [w178]
                  tunnel: [w173] -> w170 mode=indexing
                  tunnel: w168 -> [w177]
                  tunnel: w166 -> [w172] mode=indexing
                  n49 = Search 1D Array(1D array=w177, element=w172) -> (index of element=w176:i32)  [unwired: 1 in]
                  n50 = Search 1D Array(1D array=w178, element=w172) -> (index of element=w179:i32)  [unwired: 1 in]
                  n51 = Greater Or Equal To 0?(x=w176) -> (x >= 0?=w174:bool)
                  n52 = Greater Or Equal To 0?(x=w179) -> (x >= 0?=w175:bool)
                  n53 = Or(x=w174, y=w175) -> (x .or. y?=w173:bool)
                }
                n54 = And Array Elements(Boolean array=w170) -> (logical AND=w164:bool)
                n55 = Or(x=w164, y=w165) -> (x .or. y?=w162:bool)
              }
              frame Enabled {
              }
            }
            n56 = for {
              tunnel: w160 -> [w200] mode=indexing
              tunnel: w150 -> [w198]
              tunnel: [w191] -> w161 mode=indexing
              tunnel: w151 -> [w197]
              n57 = Unbundle By Name(w200) -> ("ClassName"=w196:string)
              n58 = To Lower Case(string=w196) -> (all lower case string=w195:string)
              n59 = Search 1D Array(1D array=w197, element=w195) -> (index of element=w194:i32)  [unwired: 1 in]
              n60 = Search 1D Array(1D array=w198, element=w195) -> (index of element=w199:i32)  [unwired: 1 in]
              n61 = Greater Or Equal To 0?(x=w194) -> (x >= 0?=w192:bool)
              n62 = Greater Or Equal To 0?(x=w199) -> (x >= 0?=w193:bool)
              n63 = Or(x=w192, y=w193) -> (x .or. y?=w191:bool)
            }
            n64 = Empty Array?(array=w160) -> (empty?=w158:bool)
            n65 = And Array Elements(Boolean array=w161) -> (logical AND=w159:bool)
            n66 = Or(x=w159, y=w158) -> (x .or. y?=w149:bool)
            n67 = Compound Arithmetic op=AND(w149, w148) -> (w147:bool)
            n68 = Not(x=w147) -> (.not. x?=w155:bool)
            n69 = case shown="True" w147 {
              tunnel: w154 -> [w187 w190]
              tunnel: w157 -> [_ w189]
              tunnel: [w187 w188] -> w156
              frame False {
              }
              frame True {
                n70 = Build Array (concatenate)(w190, w189) -> (w188:string[])
              }
            }
          }
          n71 = Array Size(array=w142) -> (size(s)=w140:i32)
          n72 = Array Size(array=w141) -> (size(s)=w139:i32)
          n73 = Empty Array?(array=w142) -> (empty?=w143:bool)
          n74 = Equal?(x=w140, y=w139) -> (x = y?=w138:bool)
          n75 = Or(x=w143, y=w138) -> (x .or. y?=w137:bool)
        }
        n76 = for {
          tunnel: w122 -> [w134] mode=indexing
          tunnel: [w133] -> w121 mode=indexing
          n77 = Unbundle By Name(w134) -> ("ClassName"=w133:string)
        }
        n78 = Build Array (concatenate)(w124, w121) -> (w123:string[])
        n79 = Bundle By Name(cluster=w130, "ClassesToCreate"=w123) -> (w128:T21)
      }
      frame "SortStructs" {
        n80 = Unbundle By Name(w213) -> ("EnumsToCreate"=w209:string[], "ClassesToCreate"=w208:string[], "StructsToCreate"=w212:string[], "ClassesStart"=w201:T11[])
        n81 = while {
          shift-right: [w228] -> w204
          shift-left: w212 -> [w229]
          shift-right: [w221] -> w205
          shift-left: w201 -> [w227]
          tunnel: w210 -> [w224]
          tunnel: w209 -> [w223]
          tunnel: w208 -> [w222]
          shift-right: [w218] -> _
          shift-left: 0 -> [w219]
          stop <- w225 stop-if-true
          n82 = for {
            tunnel: w227 -> [w234] mode=indexing
            shift-right: [w235] -> w228
            shift-left: w229 -> [w240]
            tunnel: w224 -> [w239]
            tunnel: w223 -> [w237]
            tunnel: w222 -> [w236]
            tunnel: [w231] -> w220 mode=indexing
            tunnel: [w233] -> w221 mode=indexing
            n83 = Unbundle By Name(w234) -> ("ClassName"=w238:string, "Structs"=w232:T1[])
            n84 = for {
              tunnel: w232 -> [w243] mode=indexing
              tunnel: w238 -> [w253]
              shift-right: [w245] -> w235
              shift-left: w240 -> [w246]
              tunnel: w239 -> [w258]
              tunnel: w237 -> [w255]
              tunnel: w236 -> [w251]
              tunnel: [w243] -> w230 mode=indexing if=w241
              n85 = Unbundle By Name(w243) -> ("Name"=w252:string, "Items"=w259:T4[])
              n86 = Concatenate Strings(w253, ":#:" ("string"), w252) -> (w244:string)
              n87 = for {
                tunnel: w255 -> [w266] mode=indexing
                tunnel: [w264] -> w250 mode=indexing
                n88 = Match Pattern(string=w266, regular expression=":#:" ("string")) -> (after substring=w264:string)  [unwired: 1 in, 3 out]
              }
              n89 = for {
                tunnel: w246 -> [w269] mode=indexing
                tunnel: [w267] -> w256 mode=indexing
                n90 = Match Pattern(string=w269, regular expression=":#:" ("string")) -> (after substring=w267:string)  [unwired: 1 in, 3 out]
              }
              n91 = for {
                tunnel: w259 -> [w285] mode=indexing
                tunnel: w258 -> [w284]
                tunnel: [w281] -> w257 mode=indexing if=w282
                n92 = Unbundle By Name(w285) -> ("DataType"=w283:T5, "DataTypeString"=w281:string)
                n93 = Search 1D Array(1D array=w284, element=w283) -> (index of element=w286:i32)  [unwired: 1 in]
                n94 = Greater Or Equal To 0?(x=w286) -> (x >= 0?=w282:bool)
              }
              n95 = Empty Array?(array=w257) -> (empty?=w247:bool)
              n96 = for {
                tunnel: w256 -> [w280]
                tunnel: w257 -> [w277] mode=indexing
                tunnel: w251 -> [w279]
                tunnel: w250 -> [w278]
                tunnel: [w270] -> w249 mode=indexing
                n97 = Search 1D Array(1D array=w278, element=w277) -> (index of element=w274:i32)  [unwired: 1 in]
                n98 = Search 1D Array(1D array=w279, element=w277) -> (index of element=w275:i32)  [unwired: 1 in]
                n99 = Search 1D Array(1D array=w280, element=w277) -> (index of element=w276:i32)  [unwired: 1 in]
                n100 = Greater Or Equal To 0?(x=w274) -> (x >= 0?=w272:bool)
                n101 = Greater Or Equal To 0?(x=w275) -> (x >= 0?=w273:bool)
                n102 = Greater Or Equal To 0?(x=w276) -> (x >= 0?=w271:bool)
                n103 = Compound Arithmetic op=OR(w272, w273, w271) -> (w270:bool)
              }
              n104 = And Array Elements(Boolean array=w249) -> (logical AND=w248:bool)
              n105 = Or(x=w248, y=w247) -> (x .or. y?=w242:bool)
              n106 = case shown="True" w242 {
                tunnel: [w260 w263] -> w245
                tunnel: w246 -> [w260 w262]
                tunnel: w244 -> [_ w261]
                frame False {
                }
                frame True {
                  n107 = Build Array (concatenate)(w262, w261) -> (w263:string[])
                }
              }
              n108 = Not(x=w242) -> (.not. x?=w241:bool)
            }
            n109 = Bundle By Name(cluster=w234, "Structs"=w230) -> (w233:T11)
            n110 = Array Size(array=w230) -> (size(s)=w231:i32)
          }
          n111 = Add Array Elements(numeric array=w220) -> (sum=w218:i32)
          n112 = Equal?(x=w218, y=w219) -> (x = y?=w226:bool)
          n113 = Equal To 0?(x=w218) -> (x = 0?=w217:bool)
          n114 = Or(x=w217, y=w226) -> (x .or. y?=w225:bool)
        }
        n115 = for {
          tunnel: w205 -> [w216] mode=indexing
          tunnel: [w215] -> w202 mode=indexing
          n116 = Unbundle By Name(w216) -> ("ClassName"=w215:string)
        }
        n117 = Build Array (concatenate)(w204, w202) -> (w203:string[])
        n118 = Bundle By Name(cluster=w213, "StructsToCreate"=w203) -> (w211:T21)
      }
      frame "OrderClasses" {
        n119 = Unbundle By Name(w297) -> ("ClassesToCreate"=w296:string[], "Classes"=w290:T11[], "ClassesStart"=w287:T11[])  [unwired: 2 out]
        n120 = for {
          tunnel: w287 -> [w301] mode=indexing
          tunnel: [w300] -> w292 mode=indexing
          n121 = Unbundle By Name(w301) -> ("ClassName"=w300:string)
        }
        n122 = Array Size(array=w290) -> (size(s)=w295:i32)
        n123 = Delete From Array(array=w296, length=w295, index=0) -> (array with subset deleted=w293:string[])  [unwired: 1 out]
        n124 = for {
          tunnel: w293 -> [w305] mode=indexing
          tunnel: w292 -> [w306]
          tunnel: w287 -> [w304]
          tunnel: [w302] -> w291 mode=indexing
          n125 = Search 1D Array(1D array=w306, element=w305) -> (index of element=w303:i32)  [unwired: 1 in]
          n126 = Index Array(array=w304, index=w303) -> (element=w302:T11)
        }
        n127 = Build Array (concatenate)(w290, w291) -> (w288:T11[])
        n128 = Bundle By Name(cluster=w297, "Classes"=w288) -> (w289:T21)
      }
      frame "CreateProject" {
        # "Set APP Ref to use when opening VIs from now on"
        n129 = invoke class="App" method="Project.New"(error in=w324) -> (error out=w322:errorcluster, "Project:New"=w323:refnum<vi>)  [unwired: 2 in, 1 out]
        n130 = call <vilib>:"Create Directory Recursive.vi"("directory"=w308) -> ("directory copy"=w307:path)  [unwired: 4 in, 2 out]
        n131 = for {
          N: 100 -> [_]
          tunnel: w307 -> [w327]
          tunnel: w322 -> [w326]
          tunnel: [w337] -> w310
          shift-right: [w338] -> w311
          shift-left: w323 -> [w339]
          i -> [w330]
          stop <- w334 continue-if-true
          n132 = Strip Path(path=w327) -> (name=w329:string)  [unwired: 1 out]
          n133 = case shown="Default" w330 {
            selector: w330 -> [w342 _]
            tunnel: [w340 _] -> w328
            frame Default {
              n134 = Format Into String(format string="(%d)", w342) -> (resulting string=w340:string)  [unwired: 2 in, 1 out]
            }
            frame 0 {
            }
          }
          n135 = Concatenate Strings(w329, w328, ".lvproj" ("string")) -> (w333:string)
          n136 = Build Path(base path=w327, name or relative path=w333) -> (appended path=w331:path)
          n137 = invoke class="Project" method="Save"(reference=w339, error in=w326, "Path"=w331) -> (reference out=w338:refnum<vi>, error out=w337:errorcluster)  [unwired: 1 in, 2 out]
          n138 = Unbundle By Name(w337) -> ("code"=w336:i32)
          n139 = Equal?(x=1357, y=w336) -> (x = y?=w334:bool)
        }
        n140 = invoke class="Project" method="Open Window"(reference=w311, error in=w310) -> (reference out=w313:refnum<vi>, error out=w312:errorcluster)  [unwired: 1 in, 1 out]
        n141 = property class="Project"(reference=w313, error in=w312) -> (reference out=w319:refnum<vi>, error out=w318:errorcluster, "App Ref"=w314:refnum<vi>)
        n142 = property class="Project"(reference=w319, error in=w318) -> (error out=w316:errorcluster, "My Computer"=w317:refnum<vi>)  [unwired: 1 out]
        n143 = Bundle By Name(cluster=w321, "Proj"=w319, "App"=w314, "ProjItem"=w317) -> (w320:T21)
        n144 = call <resource>:"CommonVIs_UmlOpenVIRef.vi"("error in"=w316, "AppRef"=w314) -> ("error out"=w315:errorcluster)  [unwired: 6 in, 3 out]
      }
      frame "CreateOutsideEnums" {
        n145 = Unbundle By Name(w344) -> ("ClassInfo"=w353:T20[])
        n146 = property class="Str"(reference=w348) -> (reference out=w352:refnum<vi>, "Value"=w351:string)  [unwired: 1 in, 1 out]
        n147 = for {
          tunnel: w347 -> [w377] mode=indexing
          shift-right: [w375] -> w349
          shift-left: w350 -> [w376]
          shift-right: [w365] -> w345
          shift-left: w353 -> [w367]
          tunnel: w352 -> [w359]
          tunnel: w351 -> [w358]
          tunnel: w346 -> [w356]
          n148 = Unbundle By Name(w377) -> ("Name"=w357:string, "Items"=w371:string[], "Documentation"=w372:string)  [unwired: 4 out]
          n149 = for {
            tunnel: w371 -> [w379] mode=indexing
            tunnel: T4 {"Name"="", "DataType"=enum."UINT8", "ArrayDim"=0, "CtrlPath"=path "", "DataTypeString"="", "AccessScope"=enum."public", "InitialData"=variant} -> [w380]
            tunnel: [w378] -> w369 mode=indexing
            n150 = Bundle By Name(cluster=w380, "Name"=w379) -> (w378:T4)
          }
          n151 = Concatenate Strings(w357, ".ctl" ("string")) -> (w363:string)
          n152 = Build Path(base path=w356, name or relative path=w363) -> (appended path=w362:path)
          n153 = call <resource>:"ReversedEngineering UpdateAttributes.vi"("ClassPath/LvClassRef"=w362, "NewAttributes"=w357, "ClassInfo"=w367, "error in (no error)"=w376, "Don't Prompt (False)"=TRUE, "Attributes"=w369, "Stereotype"="ENUM" ("regular expression"), "Ctl-Description"=w372) -> ("CtlPath"=w368:path, "error out"=w375:errorcluster)  [unwired: 9 in, 1 out]
          n154 = Format Into String(format string=" : %s", initial string=w358, w357) -> (resulting string=w361:string)  [unwired: 1 in, 1 out]
          n155 = Bundle(cluster=T20 {"ClassNamn"="", "ClassPath"=path "", "InterfaceClass"=FALSE} ("Cluster"), "ClassNamn"=w357, "ClassPath"=w368) -> (w366:T20)  [unwired: 1 in]
          n156 = property class="Str"(reference=w359, "Value"=w361) -> ()  [unwired: 1 in, 2 out]
          n157 = Build Array (concatenate)(w367, w366) -> (w365:T20[])
        }
        n158 = Bundle By Name(cluster=w344, "ClassInfo"=w345) -> (w343:T21)
      }
      frame "CreateClasses" {
        w392 = path[] []
        w393 = string[] []
        n159 = Unbundle By Name(w396) -> ("ProjItem"=w389:refnum<vi>, "Classes"=w395:T11[], "ClassInfo"=w381:T20[])
        n160 = property class="Str"(reference=w384) -> (reference out=w382:refnum<vi>, "Value"=w383:string)  [unwired: 1 in, 1 out]
        n161 = for {
          tunnel: w395 -> [w429] mode=indexing
          tunnel: w394 -> [w430]
          shift-right: [w426] -> _
          shift-left: w393 -> [w422]
          shift-right: [w425] -> _
          shift-left: w392 -> [w421]
          shift-right: [w423] -> _
          shift-left: w393 -> [w418]
          shift-right: [w424] -> _
          shift-left: w392 -> [w419]
          shift-right: [w417] -> w390
          shift-left: w391 -> [w403]
          tunnel: w389 -> [w416]
          tunnel: [w400] -> w387 mode=indexing
          tunnel: [w415] -> w386 mode=indexing
          tunnel: w383 -> [w410]
          tunnel: w382 -> [w408]
          shift-right: [w405] -> w385
          shift-left: w381 -> [w404]
          n162 = Unbundle By Name(w429) -> ("ClassName"=w406:string, "ClassDocumentation"=w427:string, "ClassType"=w412:T15, "ParentClasses"=w411:T14[])
          n163 = case shown="\"Interface\"" w412 {
            tunnel: [GDSAPI_ClassTemplateType."Standard" ("ClassTemplate") GDSAPI_ClassTemplateType."Interface(By VI Server)" ("ClassTemplate")] -> w428
            tunnel: w422 -> [w457 _]
            tunnel: w406 -> [_ _]
            tunnel: w421 -> [w456 _]
            tunnel: [w455 w475] -> w420
            tunnel: w419 -> [_ w473]
            tunnel: w418 -> [_ w474]
            tunnel: w411 -> [w454 w472]
            tunnel: w403 -> [w452 w469]
            tunnel: [w452 w468] -> w402
            tunnel: [GDSAPI_ProjectIconType."BlueFull" ("ProjectIcon-Before") w467] -> w401
            tunnel: [FALSE TRUE] -> w398
            frame "Class", Default {
              n164 = for {
                tunnel: w457 -> [w465]
                tunnel: w456 -> [w464]
                tunnel: [w463] -> w455 if=w461
                tunnel: w454 -> [w460] mode=indexing
                stop <- w461 stop-if-true
                n165 = Unbundle By Name(w460) -> ("ClassName"=w459:string)
                n166 = Search 1D Array(1D array=w465, element=w459) -> (index of element=w462:i32)  [unwired: 1 in]
                n167 = Index Array(array=w464, index=w462) -> (element=w463:path)
                n168 = Greater Or Equal To 0?(x=w462) -> (x >= 0?=w461:bool)
              }
            }
            frame "Interface" {
              n169 = for {
                tunnel: w474 -> [w483]
                tunnel: w473 -> [w482]
                tunnel: [w481] -> w475 if=w479
                tunnel: w472 -> [w478] mode=indexing
                stop <- w479 stop-if-true
                n170 = Unbundle By Name(w478) -> ("ClassName"=w477:string)
                n171 = Search 1D Array(1D array=w483, element=w477) -> (index of element=w480:i32)  [unwired: 1 in]
                n172 = Index Array(array=w482, index=w480) -> (element=w481:path)
                n173 = Greater Or Equal To 0?(x=w480) -> (x >= 0?=w479:bool)
              }
              n174 = call <resource>:"GDSAPI_SetClassOptions.vi"("SetAction(Set All)"=GDSAPI_SetClassOptionsAction."Set Project Icon Type", "error in (no error)"=w469, "ProjectIconType"=GDSAPI_ProjectIconType."Interface") -> ("error out"=w468:errorcluster, "ProjectIcon-Before"=w467:T25)  [unwired: 5 in, 2 out]
            }
          }
          n175 = Bundle By Name(cluster=T23 {"ClassProvider"=enum."GOOP-3(By reference)", "NewClassFolder"=path "", "ParentLvClassFilePath"=path "", "ClassName"="", "ClassDescription"="", "ClassTemplate"=enum."Standard"} ("CreateClassType"), "ClassProvider"=w430, "ParentLvClassFilePath"=w420, "ClassName"=w406, "ClassDescription"=w427, "ClassTemplate"=w428) -> (w431:T23)
          n176 = Format Into String(format string=" : %s", initial string=w410, w406) -> (resulting string=w409:string)  [unwired: 1 in, 1 out]
          n177 = property class="Str"(reference=w408, "Value"=w409) -> ()  [unwired: 1 in, 2 out]
          n178 = call <resource>:"GDSAPI_CreateClass.vi"("KeepLvClassRefOpen(False)"=TRUE, "error in (no error)"=w402, "CreateClassType"=w431, "ProjectItemToCraeteClassUnder"=w416) -> ("error out"=w417:errorcluster, "LVClassLibraryRefnum"=w415:refnum<vi>, "LvClassFileOut"=w400:path)  [unwired: 5 in]
          n179 = case shown="\"Interface\"" w412 {
            tunnel: w422 -> [w441 w450]
            tunnel: [w441 w449] -> w426
            tunnel: w406 -> [w435 w448]
            tunnel: [w442 w447] -> w425
            tunnel: w421 -> [w442 w446]
            tunnel: w400 -> [w436 w445]
            tunnel: w418 -> [w440 w444]
            tunnel: [w438 w444] -> w423
            tunnel: [w437 w443] -> w424
            tunnel: w419 -> [w439 w443]
            tunnel: w401 -> [w433 _]
            frame "Interface" {
              n180 = Build Array (concatenate)(w440, w435) -> (w438:string[])
              n181 = Build Array (concatenate)(w439, w436) -> (w437:path[])
              n182 = call <resource>:"GDSAPI_SetClassOptions.vi"("SetAction(Set All)"=GDSAPI_SetClassOptionsAction."Set Project Icon Type", "ProjectIconType"=w433) -> ()  [unwired: 6 in, 4 out]
            }
            frame "Class", Default {
              n183 = Build Array (concatenate)(w450, w448) -> (w449:string[])
              n184 = Build Array (concatenate)(w446, w445) -> (w447:path[])
            }
          }
          n185 = Bundle(cluster=T20 {"ClassNamn"="", "ClassPath"=path "", "InterfaceClass"=FALSE} ("Cluster"), "ClassNamn"=w406, "ClassPath"=w400, "InterfaceClass"=w398) -> (w414:T20)
          n186 = Build Array (concatenate)(w404, w414) -> (w405:T20[])
        }
        n187 = Bundle By Name(cluster=w396, "ClassPath"=w387, "ClassRefs"=w386, "ClassInfo"=w385) -> (w388:T21)
      }
      frame "CreateEnums" {
        n188 = Unbundle By Name(w495) -> ("ClassRefs"=w492:refnum<vi>[], "ClassPath"=w493:path[], "Classes"=w494:T11[], "ClassInfo"=w491:T20[])
        n189 = property class="Str"(reference=w486) -> (reference out=w485:refnum<vi>, "Value"=w484:string)  [unwired: 1 in, 1 out]
        n190 = for {
          tunnel: w494 -> [w507] mode=indexing
          tunnel: w493 -> [w505] mode=indexing
          tunnel: w492 -> [w504] mode=indexing
          shift-right: [w502] -> w487
          shift-left: w488 -> [w503]
          shift-right: [w500] -> w489
          shift-left: w491 -> [w501]
          tunnel: w485 -> [w499]
          tunnel: w484 -> [w498]
          n191 = Unbundle By Name(w507) -> ("Enums"=w506:T6[], "ClassName"=w497:string)
          n192 = for {
            tunnel: w506 -> [w532] mode=indexing
            tunnel: w505 -> [w519]
            tunnel: w504 -> [_]
            shift-right: [w530] -> w502
            shift-left: w503 -> [w531]
            shift-right: [w520] -> w500
            shift-left: w501 -> [w522]
            tunnel: w499 -> [w512]
            tunnel: w498 -> [w511]
            tunnel: w497 -> [w510]
            n193 = Unbundle By Name(w532) -> ("Name"=w509:string, "Items"=w526:string[], "Documentation"=w527:string)  [unwired: 4 out]
            n194 = Strip Path(path=w519) -> (stripped path=w517:path)  [unwired: 1 out]
            n195 = for {
              tunnel: w526 -> [w534] mode=indexing
              tunnel: T4 {"Name"="", "DataType"=enum."UINT8", "ArrayDim"=0, "CtrlPath"=path "", "DataTypeString"="", "AccessScope"=enum."public", "InitialData"=variant} -> [w535]
              tunnel: [w533] -> w524 mode=indexing
              n196 = Bundle By Name(cluster=w535, "Name"=w534) -> (w533:T4)
            }
            n197 = Concatenate Strings(w509, ".ctl" ("string")) -> (w516:string)
            n198 = Build Path(base path=w517, name or relative path=w516) -> (appended path=w515:path)
            n199 = call <resource>:"ReversedEngineering UpdateAttributes.vi"("ClassPath/LvClassRef"=w515, "NewAttributes"=w509, "ClassInfo"=w522, "error in (no error)"=w531, "Don't Prompt (False)"=TRUE, "Attributes"=w524, "Stereotype"="ENUM" ("regular expression"), "Ctl-Description"=w527) -> ("CtlPath"=w523:path, "error out"=w530:errorcluster)  [unwired: 9 in, 1 out]
            n200 = Format Into String(format string=" : %s", initial string=w511, w510) -> (resulting string=w514:string)  [unwired: 1 in, 1 out]
            n201 = Bundle(cluster=T20 {"ClassNamn"="", "ClassPath"=path "", "InterfaceClass"=FALSE} ("Cluster"), "ClassNamn"=w509, "ClassPath"=w523) -> (w521:T20)  [unwired: 1 in]
            n202 = property class="Str"(reference=w512, "Value"=w514) -> ()  [unwired: 1 in, 2 out]
            n203 = Build Array (concatenate)(w522, w521) -> (w520:T20[])
          }
        }
        n204 = Bundle By Name(cluster=w495, "ClassInfo"=w489) -> (w490:T21)
      }
      frame "CreateOusideStructs" {
        n205 = Unbundle By Name(w547) -> ("ClassInfo"=w546:T20[])  [unwired: 3 out]
        n206 = property class="Str"(reference=w541) -> (reference out=w540:refnum<vi>, "Value"=w539:string)  [unwired: 1 in, 1 out]
        n207 = for {
          shift-right: [w567] -> w542
          shift-left: w543 -> [w568]
          shift-right: [w560] -> w544
          shift-left: w546 -> [w562]
          tunnel: w540 -> [w553]
          tunnel: w539 -> [w552]
          tunnel: w537 -> [w551] mode=indexing
          tunnel: w536 -> [w550]
          n208 = Unbundle By Name(w551) -> ("Name"=w549:string, "Items"=w559:T4[], "Documentation"=w564:string)  [unwired: 2 out]
          n209 = Concatenate Strings(w549, ".ctl" ("string")) -> (w557:string)
          n210 = Build Path(base path=w550, name or relative path=w557) -> (appended path=w556:path)
          n211 = Format Into String(format string=" : %s", initial string=w552, w549) -> (resulting string=w555:string)  [unwired: 1 in, 1 out]
          n212 = property class="Str"(reference=w553, "Value"=w555) -> ()  [unwired: 1 in, 2 out]
          n213 = call <resource>:"ReversedEngineering UpdateAttributes.vi"("ClassPath/LvClassRef"=w556, "NewAttributes"=w549, "ClassInfo"=w562, "error in (no error)"=w568, "Don't Prompt (False)"=TRUE, "Attributes"=w559, "Stereotype"="STRUCT" ("regular expression"), "Ctl-Description"=w564) -> ("CtlPath"=w563:path, "error out"=w567:errorcluster)  [unwired: 9 in, 1 out]
          n214 = Bundle(cluster=T20 {"ClassNamn"="", "ClassPath"=path "", "InterfaceClass"=FALSE} ("Cluster"), "ClassNamn"=w549, "ClassPath"=w563) -> (w561:T20)  [unwired: 1 in]
          n215 = Build Array (concatenate)(w562, w561) -> (w560:T20[])
        }
        n216 = Bundle By Name(cluster=w547, "ClassInfo"=w544) -> (w545:T21)
      }
      frame "CreateStruct" {
        n217 = Unbundle By Name(w581) -> ("ClassRefs"=w578:refnum<vi>[], "ClassPath"=w579:path[], "Classes"=w580:T11[], "ClassInfo"=w577:T20[])
        n218 = property class="Str"(reference=w571) -> (reference out=w570:refnum<vi>, "Value"=w569:string)  [unwired: 1 in, 1 out]
        n219 = for {
          tunnel: w580 -> [w592] mode=indexing
          tunnel: w579 -> [w590] mode=indexing
          tunnel: w578 -> [w589] mode=indexing
          shift-right: [w587] -> w573
          shift-left: w574 -> [w588]
          shift-right: [w585] -> w575
          shift-left: w577 -> [w586]
          tunnel: w570 -> [w584]
          tunnel: w569 -> [w583]
          n220 = Unbundle By Name(w592) -> ("Structs"=w591:T1[], "ClassName"=w582:string)
          n221 = for {
            tunnel: w591 -> [w615] mode=indexing
            tunnel: w590 -> [w601]
            tunnel: w589 -> [_]
            shift-right: [w613] -> w587
            shift-left: w588 -> [w614]
            shift-right: [w606] -> w585
            shift-left: w586 -> [w608]
            tunnel: w584 -> [w597]
            tunnel: w583 -> [w596]
            tunnel: w582 -> [w594]
            n222 = Unbundle By Name(w615) -> ("Name"=w595:string, "Items"=w605:T4[], "Documentation"=w610:string)  [unwired: 2 out]
            n223 = Strip Path(path=w601) -> (stripped path=w603:path)  [unwired: 1 out]
            n224 = Concatenate Strings(w595, ".ctl" ("string")) -> (w602:string)
            n225 = Build Path(base path=w603, name or relative path=w602) -> (appended path=w600:path)
            n226 = Format Into String(format string=" : %s", initial string=w596, w594) -> (resulting string=w599:string)  [unwired: 1 in, 1 out]
            n227 = property class="Str"(reference=w597, "Value"=w599) -> ()  [unwired: 1 in, 2 out]
            n228 = call <resource>:"ReversedEngineering UpdateAttributes.vi"("ClassPath/LvClassRef"=w600, "NewAttributes"=w595, "ClassInfo"=w608, "error in (no error)"=w614, "Don't Prompt (False)"=TRUE, "Attributes"=w605, "Stereotype"="STRUCT" ("regular expression"), "Ctl-Description"=w610) -> ("CtlPath"=w609:path, "error out"=w613:errorcluster)  [unwired: 9 in, 1 out]
            n229 = Bundle(cluster=T20 {"ClassNamn"="", "ClassPath"=path "", "InterfaceClass"=FALSE} ("Cluster"), "ClassNamn"=w595, "ClassPath"=w609) -> (w607:T20)  [unwired: 1 in]
            n230 = Build Array (concatenate)(w608, w607) -> (w606:T20[])
          }
        }
        n231 = Bundle By Name(cluster=w581, "ClassInfo"=w575) -> (w576:T21)
      }
      frame "UpdateAttribute" {
        n232 = Unbundle By Name(w624) -> ("ClassRefs"=w625:refnum<vi>[], "ClassPath"=w626:path[], "Classes"=w627:T11[], "ClassInfo"=w621:T20[])
        n233 = property class="Str"(reference=w620) -> (reference out=w619:refnum<vi>, "Value"=w618:string)  [unwired: 1 in, 1 out]
        n234 = for {
          tunnel: w627 -> [w633] mode=indexing
          tunnel: w626 -> [_] mode=indexing
          tunnel: w625 -> [w643] mode=indexing
          shift-right: [w641] -> w622
          shift-left: w623 -> [w642]
          tunnel: w621 -> [w640]
          tunnel: w619 -> [w636]
          tunnel: w618 -> [w634]
          tunnel: [w629] -> w616 mode=indexing
          n235 = Unbundle By Name(w633) -> ("Attributes"=w632:T4[])
          n236 = Unbundle By Name(w633) -> ("Methods"=w631:T12[], "ClassName"=w635:string)
          n237 = Format Into String(format string=" : %s", initial string=w634, w635) -> (resulting string=w638:string)  [unwired: 1 in, 1 out]
          n238 = call <resource>:"ReversedEngineering UpdateAttributes.vi"("ClassPath/LvClassRef"=w643, "ClassInfo"=w640, "error in (no error)"=w642, "Don't Prompt (False)"=TRUE, "Attributes"=w632) -> ("error out"=w641:errorcluster)  [unwired: 12 in, 2 out]
          n239 = property class="Str"(reference=w636, "Value"=w638) -> ()  [unwired: 1 in, 2 out]
          n240 = for {
            tunnel: w632 -> [w648] mode=indexing
            shift-right: [w644] -> w630
            shift-left: w631 -> [w645]
            n241 = Unbundle By Name(w648) -> ("AccessScope"=w647:T2, "Name"=w646:string)
            n242 = case shown="\"public\"" w647 {
              tunnel: w646 -> [w651 _]
              tunnel: w645 -> [w653 w667]
              tunnel: [w659 w667] -> w644
              frame "public" {
                w655 = TRUE
                n243 = for {
                  tunnel: w653 -> [w666] mode=indexing
                  tunnel: [w665] -> w652 mode=indexing
                  n244 = Unbundle By Name(w666) -> ("MethodName"=w665:string)
                }
                n245 = Search 1D Array(1D array=w652, element=w651) -> (index of element=w650:i32)  [unwired: 1 in]
                n246 = Greater Or Equal To 0?(x=w650) -> (x >= 0?=w649:bool)
                n247 = Format Into String(format string="Attribute %s is public, therefor accessory methods have been created." ("regular expression"), w651) -> (resulting string=w657:string)  [unwired: 2 in, 1 out]
                n248 = Bundle By Name(cluster=T12 {"ReturnType"={"Name"="", "DataType"=enum."UINT8", "ArrayDim"=0, "CtrlPath"=path "", "DataTypeString"="", "AccessScope"=enum."public", "InitialData"=variant}, "MethodName"="", "AccessScope"=enum."public", "Modifiers"=[], "MethodDocumentation"="", "MethodContent"="", "MethodArguments"=[], "GetProperty"={"Active"=FALSE, "AccessScope"=enum."public", "Code"=""}, "SetProperty"={"Active"=FALSE, "AccessScope"=enum."public", "Code"=""}}, "MethodName"=w651, "AccessScope"=GDSString_AccessScopeModifierType."public", "MethodDocumentation"=w657, "GetProperty.Active"=w655, "SetProperty.Active"=w655) -> (w660:T12)
                n249 = case shown="True" w649 {
                  tunnel: w660 -> [w663 _]
                  tunnel: [w662 w664] -> w659
                  tunnel: w653 -> [w661 w664]
                  frame False {
                    n250 = Build Array (concatenate)(w663, w661) -> (w662:T12[])
                  }
                  frame True {
                  }
                }
              }
              frame Default {
              }
            }
          }
          n251 = Bundle By Name(cluster=w633, "Methods"=w630) -> (w629:T11)
        }
        n252 = Bundle By Name(cluster=w624, "Classes"=w616) -> (w617:T21)
      }
      frame "UpdateParentClassTypes" {
        n253 = Unbundle By Name(w669) -> ("ClassPath"=w676:path[], "Classes"=w668:T11[])
        n254 = for {
          tunnel: [w679] -> w675 mode=indexing
          tunnel: [w678] -> w674 mode=indexing
          tunnel: w668 -> [w677] mode=indexing
          n255 = Unbundle By Name(w677) -> ("ClassName"=w679:string, "ClassType"=w678:T15)
        }
        n256 = for {
          tunnel: w676 -> [_] mode=indexing
          tunnel: w668 -> [w682] mode=indexing
          tunnel: w675 -> [w685]
          tunnel: w674 -> [w684]
          tunnel: [w680] -> w672 mode=indexing
          n257 = Unbundle By Name(w682) -> ("ParentClasses"=w683:T14[])  [unwired: 1 out]
          n258 = Unbundle By Name(w682) -> ()  [unwired: 1 out]
          n259 = for {
            tunnel: w683 -> [w693] mode=indexing
            tunnel: w685 -> [w691]
            tunnel: w684 -> [w688]
            tunnel: [w692] -> w681 mode=indexing
            n260 = Unbundle By Name(w693) -> ("ClassName"=w690:string, "ClassType"=w686:T15)
            n261 = Search 1D Array(1D array=w691, element=w690) -> (index of element=w689:i32)  [unwired: 1 in]
            n262 = case shown="-1" w689 {
              selector: w689 -> [w695 _]
              tunnel: w688 -> [w696 _]
              tunnel: [w694 w697] -> w687
              tunnel: w686 -> [_ w699]
              frame 0, Default {
                n263 = Index Array(array=w696, index=w695) -> (element=w694:T15)
              }
              frame -1 {
                n264 = Equal?(x=w699, y=GDSString_ClassType."Undefined") -> (x = y?=w700:bool)
                n265 = Select(t=GDSString_ClassType."Class" ("y"), s=w700, f=w699) -> (s? t:f=w697:T15)
              }
            }
            n266 = Bundle By Name(cluster=w693, "ClassType"=w687) -> (w692:T14)
          }
          n267 = Bundle By Name(cluster=w682, "ParentClasses"=w681) -> (w680:T11)
        }
        n268 = Bundle By Name(cluster=w669, "Classes"=w672) -> (w671:T21)
      }
      frame "UpdateMethodTypes" {
        n269 = Unbundle By Name(w703) -> ("ClassPath"=w709:path[], "Classes"=w708:T11[], "ClassInfo"=w702:T20[])
        n270 = for {
          tunnel: w709 -> [_] mode=indexing
          tunnel: w708 -> [w712] mode=indexing
          tunnel: w702 -> [w714]
          tunnel: [w710] -> w706 mode=indexing
          n271 = Unbundle By Name(w712) -> ("Methods"=w713:T12[])  [unwired: 1 out]
          n272 = Unbundle By Name(w712) -> ()  [unwired: 1 out]
          n273 = for {
            tunnel: w713 -> [w721] mode=indexing
            tunnel: w714 -> [w722]
            tunnel: [w719] -> w711 mode=indexing
            n274 = Unbundle By Name(w721) -> ("ReturnType"=w716:T4, "MethodArguments"=w723:T4[])
            n275 = for {
              tunnel: w723 -> [w733] mode=indexing
              tunnel: w722 -> [w732]
              tunnel: [w731] -> w720 mode=indexing
              n276 = call <resource>:"CommonVIs_UpdateAttributeCtrlPath.vi"("ClassInfo"=w732, "DataType in"=w733) -> ("DataType out"=w731:T4)  [unwired: 9 in]
            }
            n277 = Unbundle By Name(w716) -> ("Name"=w715:string)
            n278 = call <resource>:"CommonVIs_UpdateAttributeCtrlPath.vi"("ClassInfo"=w722, "DataType in"=w716) -> ("DataType out"=w717:T4)  [unwired: 9 in]
            n279 = case shown="Default" w715 {
              selector: w715 -> [_ w728]
              tunnel: [w724 w730] -> w718
              tunnel: w717 -> [w724 w729]
              frame Default {
              }
              frame "" {
                n280 = Unbundle By Name(w729) -> ("DataType"=w726:T5)
                n281 = Format Into String(format string="%s Return(%s)", w728, w726) -> (resulting string=w725:string)  [unwired: 2 in, 1 out]
                n282 = Bundle By Name(cluster=w729, "Name"=w725) -> (w730:T4)
              }
            }
            n283 = Bundle By Name(cluster=w721, "ReturnType"=w718, "MethodArguments"=w720) -> (w719:T12)
          }
          n284 = Bundle By Name(cluster=w712, "Methods"=w711) -> (w710:T11)
        }
        n285 = Bundle By Name(cluster=w703, "Classes"=w706) -> (w705:T21)
      }
      frame "UpdateConstructors" {
        n286 = Unbundle By Name(w738) -> ("ClassPath"=w742:path[], "Classes"=w741:T11[], "ClassRefs"=w736:refnum<vi>[])
        n287 = for {
          tunnel: w742 -> [_] mode=indexing
          tunnel: w741 -> [w756] mode=indexing
          tunnel: [w754] -> w740 mode=indexing
          tunnel: w736 -> [w753] mode=indexing
          shift-right: [w743] -> w734
          shift-left: w735 -> [w751]
          n288 = Unbundle By Name(w756) -> ("ClassName"=w750:string, "Methods"=w757:T12[])
          n289 = call <resource>:"GDSLvClass_GetClassMethod.vi"("Class Refnum In"=w753, "VINames"=string[] ["Create", "Init"], "error in (no error)"=w751) -> ("ViPaths"=w747:path[], "error out"=w743:errorcluster)  [unwired: 13 in, 2 out]
          n290 = for {
            tunnel: w757 -> [w786] mode=indexing
            tunnel: [w786] -> w755 mode=indexing if=w784
            tunnel: w750 -> [w787]
            tunnel: [w786] -> w749 mode=indexing if=w785
            n291 = Unbundle By Name(w786) -> ("MethodName"=w788:string)
            n292 = Equal?(x=w787, y=w788) -> (x = y?=w785:bool)
            n293 = Not(x=w785) -> (.not. x?=w784:bool)
          }
          n294 = for {
            tunnel: w747 -> [w758] mode=indexing
            tunnel: [w759] -> w745
            tunnel: [w758] -> w744
            stop <- w759 continue-if-true
            n295 = Empty String/Path?(string/path=w758) -> (empty?=w759:bool)
          }
          n296 = Empty Array?(array=w749) -> (empty?=w748:bool)
          n297 = Or(x=w748, y=w745) -> (x .or. y?=w746:bool)
          n298 = case shown="False" w746 {
            tunnel: w756 -> [w778 w783]
            tunnel: w755 -> [w777 _]
            tunnel: [w776 w783] -> w754
            tunnel: w749 -> [w774 _]
            tunnel: w744 -> [w761 _]
            frame False {
              w766 = "%s" ("format string")
              w767 = "\n\n" ("delimiter (Tab)")
              n299 = for {
                tunnel: w774 -> [w782] mode=indexing
                tunnel: [w782] -> w775
                tunnel: [w781] -> w771 mode=concatenating
                tunnel: [w780] -> w770 mode=indexing
                tunnel: [w779] -> w768 mode=indexing
                n300 = Unbundle By Name(w782) -> ("MethodArguments"=w781:T4[], "MethodDocumentation"=w780:string, "MethodContent"=w779:string)
              }
              n301 = call <vilib>:"Get File Extension.vi"("file"=w761) -> ("filename without extension"=w760:string)  [unwired: 6 in, 4 out]
              n302 = Array To Spreadsheet String(delimiter (Tab)=w767, array=w770, 3:w766) -> (spreadsheet string=w769:string)
              n303 = Array To Spreadsheet String(delimiter (Tab)=w767, array=w768, 3:w766) -> (spreadsheet string=w765:string)
              n304 = call <vilib>:"Trim Whitespace.vi"("string"=w769) -> ("trimmed string"=w764:string)  [unwired: 1 in]
              n305 = call <vilib>:"Trim Whitespace.vi"("string"=w765) -> ("trimmed string"=w763:string)  [unwired: 1 in]
              n306 = Bundle By Name(cluster=w775, "ReturnType"=T4 {"Name"="", "DataType"=enum."void", "ArrayDim"=0, "CtrlPath"=path "", "DataTypeString"="", "AccessScope"=enum."public", "InitialData"=variant}, "MethodArguments"=w771, "MethodDocumentation"=w764, "MethodContent"=w763, "MethodName"=w760) -> (w762:T12)
              n307 = Build Array (concatenate)(w777, w762) -> (w773:T12[])
              n308 = Bundle By Name(cluster=w778, "Methods"=w773) -> (w776:T11)
            }
            frame True {
            }
          }
        }
        n309 = Bundle By Name(cluster=w738, "Classes"=w740) -> (w739:T21)
      }
      frame "UpdateDestructors" {
        n310 = Unbundle By Name(w793) -> ("ClassPath"=w797:path[], "Classes"=w796:T11[], "ClassRefs"=w791:refnum<vi>[])
        n311 = for {
          tunnel: w797 -> [_] mode=indexing
          tunnel: w796 -> [w811] mode=indexing
          tunnel: [w809] -> w795 mode=indexing
          tunnel: w791 -> [w808] mode=indexing
          shift-right: [w798] -> w789
          shift-left: w790 -> [w806]
          n312 = Unbundle By Name(w811) -> ("ClassName"=w805:string, "Methods"=w812:T12[])
          n313 = for {
            tunnel: w812 -> [w848] mode=indexing
            tunnel: [w848] -> w810 mode=indexing if=w847
            tunnel: w805 -> [w846]
            tunnel: [w848] -> w804 mode=indexing if=w841
            n314 = Unbundle By Name(w848) -> ("MethodName"=w844:string)
            n315 = Format Into String(format string="~%s", w846) -> (resulting string=w845:string)  [unwired: 2 in, 1 out]
            n316 = Equal?(x="finalize", y=w844) -> (x = y?=w843:bool)
            n317 = Equal?(x=w845, y=w844) -> (x = y?=w842:bool)
            n318 = Or(x=w843, y=w842) -> (x .or. y?=w841:bool)
            n319 = Not(x=w841) -> (.not. x?=w847:bool)
          }
          n320 = call <resource>:"GDSLvClass_GetClassMethod.vi"("Class Refnum In"=w808, "VINames"=string[] ["Destroy", "CleanUp"], "error in (no error)"=w806) -> ("ViPaths"=w802:path[], "error out"=w798:errorcluster)  [unwired: 13 in, 2 out]
          n321 = for {
            tunnel: w802 -> [w813] mode=indexing
            tunnel: [w814] -> w800
            tunnel: [w813] -> w799
            stop <- w814 continue-if-true
            n322 = Empty String/Path?(string/path=w813) -> (empty?=w814:bool)
          }
          n323 = Empty Array?(array=w804) -> (empty?=w803:bool)
          n324 = Or(x=w803, y=w800) -> (x .or. y?=w801:bool)
          n325 = case shown="False" w801 {
            tunnel: w811 -> [w833 w838]
            tunnel: w810 -> [w832 _]
            tunnel: [w831 w838] -> w809
            tunnel: w804 -> [w829 _]
            tunnel: w799 -> [w816 _]
            frame False {
              w821 = "%s" ("format string")
              w822 = "\n\n" ("delimiter (Tab)")
              n326 = for {
                tunnel: w829 -> [w837] mode=indexing
                tunnel: [w837] -> w830
                tunnel: [w836] -> w826 mode=concatenating
                tunnel: [w835] -> w825 mode=indexing
                tunnel: [w834] -> w823 mode=indexing
                n327 = Unbundle By Name(w837) -> ("MethodArguments"=w836:T4[], "MethodDocumentation"=w835:string, "MethodContent"=w834:string)
              }
              n328 = call <vilib>:"Get File Extension.vi"("file"=w816) -> ("filename without extension"=w815:string)  [unwired: 6 in, 4 out]
              n329 = Array To Spreadsheet String(delimiter (Tab)=w822, array=w825, 3:w821) -> (spreadsheet string=w824:string)
              n330 = Array To Spreadsheet String(delimiter (Tab)=w822, array=w823, 3:w821) -> (spreadsheet string=w820:string)
              n331 = call <vilib>:"Trim Whitespace.vi"("string"=w824) -> ("trimmed string"=w819:string)  [unwired: 1 in]
              n332 = call <vilib>:"Trim Whitespace.vi"("string"=w820) -> ("trimmed string"=w818:string)  [unwired: 1 in]
              n333 = Bundle By Name(cluster=w830, "ReturnType"=T4 {"Name"="", "DataType"=enum."void", "ArrayDim"=0, "CtrlPath"=path "", "DataTypeString"="", "AccessScope"=enum."public", "InitialData"=variant}, "MethodArguments"=w826, "MethodDocumentation"=w819, "MethodContent"=w818, "MethodName"=w815) -> (w817:T12)
              n334 = Build Array (concatenate)(w832, w817) -> (w828:T12[])
              n335 = Bundle By Name(cluster=w833, "Methods"=w828) -> (w831:T11)
            }
            frame True {
            }
          }
        }
        n336 = Bundle By Name(cluster=w793, "Classes"=w795) -> (w794:T21)
      }
      frame "AddInterfaceMethods" {
        n337 = property class="Str"(reference=w852) -> (reference out=w851:refnum<vi>, "Value"=w850:string)  [unwired: 1 in, 1 out]
        n338 = Unbundle By Name(w853) -> ("ClassPath"=w857:path[], "Classes"=w856:T11[])  [unwired: 1 out]
        n339 = for {
          shift-right: [w867] -> w854
          shift-left: w855 -> [w868]
          tunnel: w857 -> [w859] mode=indexing
          tunnel: w856 -> [w860] mode=indexing
          tunnel: w851 -> [w863]
          tunnel: w850 -> [w862]
          n340 = Unbundle By Name(w860) -> ("Methods"=w866:T12[], "ClassName"=w861:string)
          n341 = Unbundle By Name(w860) -> ("ClassType"=w858:T15)
          n342 = case shown="\"Interface\"" w858 {
            tunnel: w868 -> [w869 w873]
            tunnel: [w869 w872] -> w867
            tunnel: w866 -> [_ w870]
            tunnel: w859 -> [_ w871]
            frame Default {
            }
            frame "Interface" {
              n343 = call <resource>:"GDSAPI_CreateMethods2.vi"("error in (no error)"=w873, "Methods"=w870, "ClassPath(*.lvclass)"=w871) -> ("error out"=w872:errorcluster)  [unwired: 7 in, 1 out]
            }
          }
          n344 = Format Into String(format string=" : %s", initial string=w862, w861) -> (resulting string=w865:string)  [unwired: 1 in, 1 out]
          n345 = property class="Str"(reference=w863, "Value"=w865) -> ()  [unwired: 1 in, 2 out]
        }
      }
      frame "AddDesignPattern" {
        # "Implement Deisgn pattern (Interface), also remove any methods that the interface-design pattern will add to the class"
        n346 = Unbundle By Name(w878) -> ("ClassPath"=w886:path[], "Classes"=w874:T11[], "ClassInfo"=w885:T20[])  [unwired: 1 out]
        n347 = property class="Str"(reference=w882) -> (reference out=w881:refnum<vi>, "Value"=w880:string)  [unwired: 1 in, 1 out]
        n348 = for {
          tunnel: w885 -> [w893] mode=indexing
          tunnel: [w892] -> w884 mode=indexing
          tunnel: [w891] -> w883 mode=indexing
          n349 = Unbundle By Name(w893) -> ("ClassNamn"=w892:string, "ClassPath"=w891:path)
        }
        n350 = for {
          tunnel: w874 -> [w890] mode=indexing
          tunnel: [w889] -> w875 mode=indexing
          n351 = Unbundle By Name(w890) -> ("ClassName"=w889:string)
        }
        n352 = for {
          shift-right: [w906] -> w879
          shift-left: w887 -> [w907]
          tunnel: w886 -> [w905] mode=indexing
          tunnel: w874 -> [w898] mode=indexing
          tunnel: w884 -> [w904]
          tunnel: w883 -> [w903]
          tunnel: w881 -> [w902]
          tunnel: w880 -> [w901]
          tunnel: [w896] -> w876 mode=indexing
          tunnel: w875 -> [w895]
          tunnel: w874 -> [w894]
          n353 = Unbundle By Name(w898) -> ("ParentClasses"=w908:T14[], "ClassName"=w900:string)
          n354 = Unbundle By Name(w898) -> ("Methods"=w899:T12[])  [unwired: 1 out]
          n355 = for {
            tunnel: w908 -> [w923] mode=indexing
            shift-right: [w920] -> w906
            shift-left: w907 -> [w921]
            tunnel: w905 -> [w919]
            tunnel: w904 -> [w918]
            tunnel: w903 -> [w916]
            tunnel: w902 -> [w915]
            tunnel: w901 -> [w914]
            tunnel: w900 -> [w913]
            shift-right: [w911] -> w897
            shift-left: w899 -> [w912]
            tunnel: w895 -> [w910]
            tunnel: w894 -> [w909]
            n356 = Unbundle By Name(w923) -> ("ClassType"=w922:T15, "ClassName"=w917:string)
            n357 = case shown="\"Interface\"" w922 {
              tunnel: w921 -> [w925 w940]
              tunnel: [w925 w939] -> w920
              tunnel: w919 -> [_ w938]
              tunnel: w918 -> [_ w937]
              tunnel: w917 -> [_ w928]
              tunnel: w916 -> [_ w936]
              tunnel: w915 -> [_ w934]
              tunnel: w914 -> [_ w933]
              tunnel: w913 -> [_ w932]
              tunnel: w912 -> [w924 w931]
              tunnel: [w924 w930] -> w911
              tunnel: w910 -> [_ w929]
              tunnel: w909 -> [_ w927]
              frame "Undefined", Default {
              }
              frame "Interface" {
                n358 = Search 1D Array(1D array=w937, element=w928) -> (index of element=w935:i32)  [unwired: 1 in]
                n359 = Search 1D Array(1D array=w929, element=w928) -> (index of element=w926:i32)  [unwired: 1 in]
                n360 = case shown="Default" w935 {
                  tunnel: w940 -> [w942 w961]
                  tunnel: [w942 w944] -> w939
                  tunnel: w938 -> [_ w943]
                  tunnel: w936 -> [_ w960]
                  tunnel: w935 -> [_ w959]
                  tunnel: w934 -> [_ w955]
                  tunnel: w933 -> [_ w954]
                  tunnel: w932 -> [_ w953]
                  tunnel: w931 -> [w941 w949]
                  tunnel: [w941 w946] -> w930
                  tunnel: w927 -> [_ w952]
                  tunnel: w926 -> [_ w951]
                  frame -1 {
                  }
                  frame Default {
                    # "Add MethodContent to the newly created Methods"
                    n361 = Index Array(array=w952, index=w951) -> (element=w950:T11)
                    n362 = Index Array(array=w960, index=w959) -> (element=w958:path)
                    n363 = Format Into String(format string=" : %s", initial string=w954, w953) -> (resulting string=w957:string)  [unwired: 1 in, 1 out]
                    n364 = Unbundle By Name(w950) -> ("Methods"=w948:T12[])
                    n365 = call <resource>:"GDSAPI_AddDeisgnPattern.vi"("error in (no error)"=w961, "InterfaceClass(*.lvclass)"=w958, "ClassPath(*.lvclass)"=w943) -> ("error out"=w945:errorcluster)  [unwired: 8 in]
                    n366 = property class="Str"(reference=w955, "Value"=w957) -> ()  [unwired: 1 in, 2 out]
                    n367 = for {
                      tunnel: w948 -> [w963] mode=indexing
                      tunnel: [w962] -> w947 mode=indexing
                      n368 = Unbundle By Name(w963) -> ("MethodName"=w962:string)
                    }
                    n369 = for {
                      tunnel: w949 -> [w971] mode=indexing
                      tunnel: w947 -> [w972]
                      tunnel: [w971] -> w946 mode=indexing if=w969
                      shift-right: [w967] -> w944
                      shift-left: w945 -> [w968]
                      tunnel: w943 -> [w966]
                      n370 = Unbundle By Name(w971) -> ("MethodName"=w965:string, "MethodContent"=w964:string)
                      n371 = Search 1D Array(1D array=w972, element=w965) -> (index of element=w970:i32)  [unwired: 1 in]
                      n372 = Less Than 0?(x=w970) -> (x < 0?=w969:bool)
                      n373 = call <resource>:"ConvertTextBasedCodeToLabVIEW_AddMethodContentToBdOfClassMethod.vi"("error in (no error)"=w968, "MethodContent"=w964, "MethodName"=w965, "ClassPath(*.lvclass)"=w966) -> ("error out"=w967:errorcluster)  [unwired: 7 in]
                    }
                  }
                }
              }
            }
          }
          n374 = Bundle By Name(cluster=w898, "Methods"=w897) -> (w896:T11)
        }
        n375 = Bundle By Name(cluster=w878, "Classes"=w876) -> (w877:T21)
      }
      frame "CreateMethods" {
        n376 = property class="Str"(reference=w976) -> (reference out=w975:refnum<vi>, "Value"=w974:string)  [unwired: 1 in, 1 out]
        n377 = Unbundle By Name(w977) -> ("ClassPath"=w981:path[], "Classes"=w980:T11[])
        n378 = for {
          shift-right: [w992] -> w978
          shift-left: w979 -> [w994]
          tunnel: w981 -> [w993] mode=indexing
          tunnel: w980 -> [w985] mode=indexing
          tunnel: w975 -> [w988]
          tunnel: w974 -> [w987]
          tunnel: w973 -> [w983]
          n379 = Unbundle By Name(w985) -> ("Methods"=w991:T12[], "ClassName"=w986:string)
          n380 = Unbundle By Name(w985) -> ("ClassType"=w984:T15)
          n381 = case shown="\"Class\", Default" w984 {
            tunnel: w994 -> [w995 w1000]
            tunnel: w993 -> [_ w999]
            tunnel: [w995 w998] -> w992
            tunnel: w991 -> [_ w997]
            tunnel: w983 -> [_ w996]
            frame "Interface" {
            }
            frame "Class", Default {
              n382 = call <resource>:"GDSAPI_CreateMethods2.vi"("PropertyMethodType"=w996, "error in (no error)"=w1000, "Methods"=w997, "ClassPath(*.lvclass)"=w999) -> ("error out"=w998:errorcluster)  [unwired: 6 in, 1 out]
            }
          }
          n383 = Format Into String(format string=" : %s", initial string=w987, w986) -> (resulting string=w990:string)  [unwired: 1 in, 1 out]
          n384 = property class="Str"(reference=w988, "Value"=w990) -> ()  [unwired: 1 in, 2 out]
        }
      }
      frame "SaveAll" {
        w1006 = TRUE ("ExcludeDependencies")
        n385 = Unbundle By Name(w1009) -> ("Proj"=w1008:refnum<vi>)  [unwired: 3 out]
        n386 = property class="Project"(reference=w1008) -> ("My Computer"=w1007:refnum<vi>)  [unwired: 1 in, 2 out]
        n387 = invoke class="TargetItem" method="Get All Descendents"(reference=w1007, "Exclude Dependencies"=w1006, "ExcludeBuilds"=w1006, "ExcludeTargets"=w1006) -> (reference out=w1001:refnum<vi>, "All Descendents"=w1003:refnum<vi>[])  [unwired: 3 in, 5 out]
        n388 = for {
          tunnel: w1003 -> [w1015] mode=indexing
          tunnel: [w1011] -> w1004
          n389 = property class="ProjectItem"(reference=w1015) -> (reference out=w1012:refnum<vi>, error out=w1011:errorcluster, "Reference"=w1013:refnum<vi>)  [unwired: 1 in]
          n390 = Not A Number/Path/Refnum?(number/path/refnum=w1013) -> (NaN/Path/Refnum?=w1014:bool)
          n391 = case shown="True" w1014 {
            tunnel: w1013 -> [w1018 _]
            tunnel: w1012 -> [_ w1022]
            frame False {
              n392 = invoke class="VI" method="Save.Instrument"(reference=w1018) -> (reference out=w1016:refnum<vi>, error out=w1017:errorcluster)  [unwired: 5 in, 4 out]
              n393 = Close Reference(reference=w1016, error in (no error)=w1017) -> ()  [unwired: 1 out]
            }
            frame True {
              w1021 = refnum<vi> refnum  # LVClassLibrary
              n394 = To More Specific Class(target class=w1021, reference=w1022) -> (specific class reference=w1019:refnum<vi>, error out=w1020:errorcluster)  [unwired: 1 in]
              n395 = case shown="No Error" w1020 {
                tunnel: w1019 -> [w1023 _]
                frame No Error {
                  n396 = invoke class="LVClassLibrary" method="Save"(reference=w1023) -> ()  [unwired: 3 in, 4 out]
                }
                frame Error {
                }
              }
            }
          }
        }
        n397 = Close Reference(reference=w1003, error in (no error)=w1004) -> (error out=w1002:errorcluster)
        n398 = Close Reference(reference=w1001, error in (no error)=w1002) -> ()  [unwired: 1 out]
      }
      frame "Done" {
        n399 = Unbundle By Name(w1047) -> ("StartTime"=w1036:timestamp, "App"=w1040:refnum<vi>, "Proj"=w1046:refnum<vi>, "ProjItem"=w1044:refnum<vi>)
        n400 = Close Reference(reference=w1044, error in (no error)=w1039) -> (error out=w1043:errorcluster)
        n401 = invoke class="Project" method="Save"(reference=w1046, error in=w1043) -> (reference out=w1042:refnum<vi>, error out=w1045:errorcluster)  [unwired: 2 in, 2 out]
        n402 = Close Reference(reference=w1042, error in (no error)=w1045) -> (error out=w1041:errorcluster)
        n403 = Close Reference(reference=w1040, error in (no error)=w1041) -> (error out=w1038:errorcluster)
        n404 = Get Date/Time In Seconds() -> (seconds since 1Jan1904=w1037:timestamp)
        n405 = Subtract(x=w1037, y=w1036) -> (x-y=w1035:dbl)
        n406 = Quotient & Remainder(x=w1035, y=60.0) -> (x-y*floor(x/y)=w1025:dbl, floor(x/y)=w1026:dbl)
        n407 = property class="Str"(reference=w1028) -> (reference out=w1030:refnum<vi>, "Value"=w1032:string)  [unwired: 1 in, 1 out]
        n408 = Format Into String(format string="Conversion completed in %d min %02d s", w1026, w1025) -> (resulting string=w1024:string)  [unwired: 2 in, 1 out]
        n409 = Concatenate Strings(w1032, "\n" ("string"), w1024) -> (w1031:string)
        n410 = property class="Str"(reference=w1030, "Value"=w1031, "Text.Scroll Position"=u32 4294967295) -> ()  [unwired: 1 in, 2 out]
      }
      frame "CloseDown", "Error", Default {
        n411 = call <resource>:"CommonVIs_UmlOpenVIRef.vi"("ProjectNameIn"="clear", "error in"=w1050) -> ("error out"=w1049:errorcluster)  [unwired: 6 in, 3 out]
      }
    }
    n412 = Unbundle By Name(w31) -> ("Classes"=→"ClassesOut":T11[])
    n413 = Equal?(x=w50, y="Exit") -> (x = y?=w48:bool)
    n414 = Select(t="Error", s=w53, f=w50) -> (s? t:f=w51:string)
  }
  "error out" <- w20
  n415 = Unbundle By Name(w6) -> ("Pattern-Before"=w5:T10)
  n416 = call <resource>:"GDSAPI_SetClassOptions.vi"("SetAction(Set All)"=GDSAPI_SetClassOptionsAction."Set Pattern Type", "PatternIn"=w5) -> ()  [unwired: 6 in, 4 out]
